vi "Gas Rack Cal UI.vi"(11 "Calling VI Ref":refnum<vi>) -> ()   [LabVIEW 2019]
uses:
  Type Defs/Units Type Def (DAQ Rack).ctl
  Type Defs/Gas Rack Channel Type Def (RIO).ctl
  Type Defs/Targets Type Def.ctl
  Type Defs/Target Cluster Type Def.ctl
  Type Defs/Setpoint Cluster Type Def.ctl
  Type Defs/Rack Version Type Def.ctl
  Type Defs/Registered System.ctl
  Type Defs/System Type.ctl
  Type Defs/TCP Data Stream Mode (PC).ctl
  <vilib>/Utility/miscctls.llb/LVRowAndColumnTypeDef.ctl
  <vilib>/Utility/file.llb/Write To Spreadsheet File (string).vi
  <vilib>/Utility/file.llb/Read From Spreadsheet File (string).vi
  <userlib>/_OpenG.lib/array/array.llb/Remove Duplicates from 1D Array (DBL)__ogtk.vi
  <userlib>/_OpenG.lib/array/array.llb/Search 1D Array (String)__ogtk.vi
  <vilib>/ptbypt/NI_PtbyPt.lvlib
  <vilib>/Analysis/NI_AALPro.lvlib
  <resource>/objmgr/daqmx.rc
  <vilib>/Utility/config.llb/NI_LVConfig.lvlib
  <vilib>/FTP/NI_FTP.lvlib
panel:
  out "RIO Found":bool
  out "Lost Connection":bool
  in  "Stop Second Loop":bool
  out "a0":dbl format="%#.4g"
  out "a2":dbl format="%#.4g"
  out "a1":dbl format="%#.4g"
  out "a3":dbl format="%#.4g"
  out "a4":dbl format="%#.4g"
  in  "App Dir":path
  in  "Load Indicator Tab":enum32{"Page 1"}(tab)
  in  "Header Tab":enum32{"Page 1", "Page 2"}(tab)
  in  "Header OK":bool
  in  "Header Cancel":bool
  in  "Header Comments":string[][](table)=[[""], [""], [""]]
  in  "Cal Standards Table":string[][](table)=[["", ""], ["", ""], ["", ""], ["", ""], ["", ""]]
  in  "Sys Cal Table":string[][](table)=[["", ""], ["", ""], ["", ""], ["", ""], ["", ""]]
  in  "Header Table 1":string[][](table)=[[""], [""], [""], [""], [""], [""], [""], [""]]
  in  "Header Table 2":string[][](table)=[[""], [""], [""], [""], [""], [""], [""]]
  in  "debug":bool=TRUE
  in  "Output Tab":enum32{"Page 1", "Page 2"}(tab)
  out "Row":i32
  in  "Main Tab":enum32{"Page 1", "Page 2"}(tab)
  in  "Channel to Cal":T1
  in  "Transfer Cal":bool
  in  "Verify Tab":enum32{"Page 1", "Page 2"}(tab)
  out "Ver Reading":dbl=0.0016 caption="reading" format="%#.4g"
  in  "Hide Devs":bool
  in  "Auto":bool
  in  "Hide Cal Values":bool
  in  "Verify Edit":bool
  in  "Verify Table":string[][](table)=[["", "0", "0"], ["", "3", "3"], ["", "6", "6"], ["", "9", "9"], ["", "12", "12"], ["", "15", "15"], ["", "", ""], ["", "", ""], ["", "", ""], ["", "", ""]]
  in  "Verify Read":bool
  in  "ms":u32=1000
  in  "avg":i32=5
  in  "Save Cal":bool
  in  "Cancel Verify":bool
  in  "Cal Tab":enum32{"Apply", "Cal"}(tab)
  in  "Cancel Cal":bool
  in  "Apply Cal":bool
  in  "Confirm Cal Point":bool
  in  "Master Value":dbl caption="cal pt" format="%#.4g"
  out "Cal Reading":dbl=0.0016 caption="reading" format="%#.4g"
  in  "4th Point Cal":bool
  out "Reading Value 4":dbl caption="reading" format="%#.4g"
  in  "Cal Value 4":dbl caption="cal pt" format="%#.4g"
  in  "5th Point Cal":bool
  out "Reading Value 5":dbl caption="reading" format="%#.4g"
  in  "Cal Value 5":dbl caption="cal pt" format="%#.4g"
  in  "Start Verification":bool
  in  "Header":bool
  out "Cal Table":string[][](table)=[["AI-00", "V", "", "", "", "", "", "", "", "", "", "", "", "", "", "", "", "", "", "", "", "", "", "", "", "", "", "", "", "", "", ""], ["AI-01", "V", "", "", "", "", "", "", "", "", "", "", "", "", "", "", "", "", "", "", "", "", "", "", "", "", "", "", "", "", "", ""], ["AI-02", "V", "", "", "", "", "", "", "", "", "", "", "", "", "", "", "", "", "", "", "", "", "", "", "", "", "", "", "", "", "", ""], ["AI-03", "V", "", "", "", "", "", "", "", "", "", "", "", "", "", "", "", "", "", "", "", "", "", "", "", "", "", "", "", "", "", ""], ["AI-04", "V", "", "", "", "", "", "", "", "", "", "", "", "", "", "", "", "", "", "", "", "", "", "", "", "", "", "", "", "", "", ""], ["AI-05", "V", "", "", "", "", "", "", "", "", "", "", "", "", "", "", "", "", "", "", "", "", "", "", "", "", "", "", "", "", "", ""], ["AI-06", "V", "", "", "", "", "", "", "", "", "", "", "", "", "", "", "", "", "", "", "", "", "", "", "", "", "", "", "", "", "", ""], ["AI-07", "V", "", "", "", "", "", "", "", "", "", "", "", "", "", "", "", "", "", "", "", "", "", "", "", "", "", "", "", "", "", ""], ["AI-08", "V", "", "", "", "", "", "", "", "", "", "", "", "", "", "", "", "", "", "", "", "", "", "", "", "", "", "", "", "", "", ""], ["AI-09", "V", "", "", "", "", "", "", "", "", "", "", "", "", "", "", "", "", "", "", "", "", "", "", "", "", "", "", "", "", "", ""], ["AI-10", "V", "", "", "", "", "", "", "", "", "", "", "", "", "", "", "", "", "", "", "", "", "", "", "", "", "", "", "", "", "", ""], ["AI-11", "V", "", "", "", "", "", "", "", "", "", "", "", "", "", "", "", "", "", "", "", "", "", "", "", "", "", "", "", "", "", ""], ["AI-12", "V", "", "", "", "", "", "", "", "", "", "", "", "", "", "", "", "", "", "", "", "", "", "", "", "", "", "", "", "", "", ""], ["AI-13", "V", "", "", "", "", "", "", "", "", "", "", "", "", "", "", "", "", "", "", "", "", "", "", "", "", "", "", "", "", "", ""], ["AI-14", "V", "", "", "", "", "", "", "", "", "", "", "", "", "", "", "", "", "", "", "", "", "", "", "", "", "", "", "", "", "", ""], ["AI-15", "V", "", "", "", "", "", "", "", "", "", "", "", "", "", "", "", "", "", "", "", "", "", "", "", "", "", "", "", "", "", ""], ["AI-16", "V", "", "", "", "", "", "", "", "", "", "", "", "", "", "", "", "", "", "", "", "", "", "", "", "", "", "", "", "", "", ""], ["AI-17", "V", "", "", "", "", "", "", "", "", "", "", "", "", "", "", "", "", "", "", "", "", "", "", "", "", "", "", "", "", "", ""], ["AI-18", "V", "", "", "", "", "", "", "", "", "", "", "", "", "", "", "", "", "", "", "", "", "", "", "", "", "", "", "", "", "", ""], ["AI-19", "V", "", "", "", "", "", "", "", "", "", "", "", "", "", "", "", "", "", "", "", "", "", "", "", "", "", "", "", "", "", ""], ["AI-20", "V", "", "", "", "", "", "", "", "", "", "", "", "", "", "", "", "", "", "", "", "", "", "", "", "", "", "", "", "", "", ""], ["AI-21", "V", "", "", "", "", "", "", "", "", "", "", "", "", "", "", "", "", "", "", "", "", "", "", "", "", "", "", "", "", "", ""], ["AI-22", "V", "", "", "", "", "", "", "", "", "", "", "", "", "", "", "", "", "", "", "", "", "", "", "", "", "", "", "", "", "", ""], ["AI-23", "V", "", "", "", "", "", "", "", "", "", "", "", "", "", "", "", "", "", "", "", "", "", "", "", "", "", "", "", "", "", ""], ["AI-24", "V", "", "", "", "", "", "", "", "", "", "", "", "", "", "", "", "", "", "", "", "", "", "", "", "", "", "", "", "", "", ""], ["AI-25", "V", "", "", "", "", "", "", "", "", "", "", "", "", "", "", "", "", "", "", "", "", "", "", "", "", "", "", "", "", "", ""], ["AI-26", "V", "", "", "", "", "", "", "", "", "", "", "", "", "", "", "", "", "", "", "", "", "", "", "", "", "", "", "", "", "", ""], ["AI-27", "V", "", "", "", "", "", "", "", "", "", "", "", "", "", "", "", "", "", "", "", "", "", "", "", "", "", "", "", "", "", ""], ["AI-28", "V", "", "", "", "", "", "", "", "", "", "", "", "", "", "", "", "", "", "", "", "", "", "", "", "", "", "", "", "", "", ""], ["AI-29", "V", "", "", "", "", "", "", "", "", "", "", "", "", "", "", "", "", "", "", "", "", "", "", "", "", "", "", "", "", "", ""], ["AI-30", "V", "", "", "", "", "", "", "", "", "", "", "", "", "", "", "", "", "", "", "", "", "", "", "", "", "", "", "", "", "", ""], ["AI-31", "V", "", "", "", "", "", "", "", "", "", "", "", "", "", "", "", "", "", "", "", "", "", "", "", "", "", "", "", "", "", ""], ["TC-00", "degF", "", "", "", "", "", "", "", "", "", "", "", "", "", "", "", "", "", "", "", "", "", "", "", "", "", "", "", "", "", ""], ["TC-01", "degF", "", "", "", "", "", "", "", "", "", "", "", "", "", "", "", "", "", "", "", "", "", "", "", "", "", "", "", "", "", ""], ["TC-02", "degF", "", "", "", "", "", "", "", "", "", "", "", "", "", "", "", "", "", "", "", "", "", "", "", "", "", "", "", "", "", ""], ["TC-03", "degF", "", "", "", "", "", "", "", "", "", "", "", "", "", "", "", "", "", "", "", "", "", "", "", "", "", "", "", "", "", ""], ["TC-04", "degF", "", "", "", "", "", "", "", "", "", "", "", "", "", "", "", "", "", "", "", "", "", "", "", "", "", "", "", "", "", ""], ["TC-05", "degF", "", "", "", "", "", "", "", "", "", "", "", "", "", "", "", "", "", "", "", "", "", "", "", "", "", "", "", "", "", ""], ["TC-06", "degF", "", "", "", "", "", "", "", "", "", "", "", "", "", "", "", "", "", "", "", "", "", "", "", "", "", "", "", "", "", ""], ["TC-07", "degF", "", "", "", "", "", "", "", "", "", "", "", "", "", "", "", "", "", "", "", "", "", "", "", "", "", "", "", "", "", ""], ["TC-08", "degF", "", "", "", "", "", "", "", "", "", "", "", "", "", "", "", "", "", "", "", "", "", "", "", "", "", "", "", "", "", ""], ["TC-09", "degF", "", "", "", "", "", "", "", "", "", "", "", "", "", "", "", "", "", "", "", "", "", "", "", "", "", "", "", "", "", ""], ["TC-10", "degF", "", "", "", "", "", "", "", "", "", "", "", "", "", "", "", "", "", "", "", "", "", "", "", "", "", "", "", "", "", ""], ["TC-11", "degF", "", "", "", "", "", "", "", "", "", "", "", "", "", "", "", "", "", "", "", "", "", "", "", "", "", "", "", "", "", ""], ["TC-12", "degF", "", "", "", "", "", "", "", "", "", "", "", "", "", "", "", "", "", "", "", "", "", "", "", "", "", "", "", "", "", ""], ["TC-13", "degF", "", "", "", "", "", "", "", "", "", "", "", "", "", "", "", "", "", "", "", "", "", "", "", "", "", "", "", "", "", ""], ["TC-14", "degF", "", "", "", "", "", "", "", "", "", "", "", "", "", "", "", "", "", "", "", "", "", "", "", "", "", "", "", "", "", ""], ["TC-15", "degF", "", "", "", "", "", "", "", "", "", "", "", "", "", "", "", "", "", "", "", "", "", "", "", "", "", "", "", "", "", ""], ["", "", "", "", "", "", "", "", "", "", "", "", "", "", "", "", "", "", "", "", "", "", "", "", "", "", "", "", "", "", "", ""]]
  out "Tank IP:":string
  in  "Start Cal":bool
  in  "1st Point Cal":bool
  out "Reading Value 1":dbl caption="Read Data" format="%#.4g"
  in  "Cal Value 1":dbl caption="Cal Point" format="%#.4g"
  in  "2nd Point Cal":bool
  out "Reading Value 2":dbl caption="reading" format="%#.4g"
  in  "Cal Value 2":dbl caption="cal pt" format="%#.4g"
  in  "Cal Unit":T2
  in  "3rd Point Cal":bool
  out "Reading Value 3":dbl caption="reading" format="%#.4g"
  in  "Cal Value 3":dbl caption="cal pt" format="%#.4g"
  in  "View Spreadsheet":bool
  # "Channel Data"
  # "System Calibration Components"
  # "Calibration Standards Used"
  # "Output Control"
  # "Enter Header Info"
  # "Calibration"
  # "Verification"
  # "Select Channel to Calibrate"
  # "Cal Spreadsheet"
  # "*Excel must be closed to return control to this app."
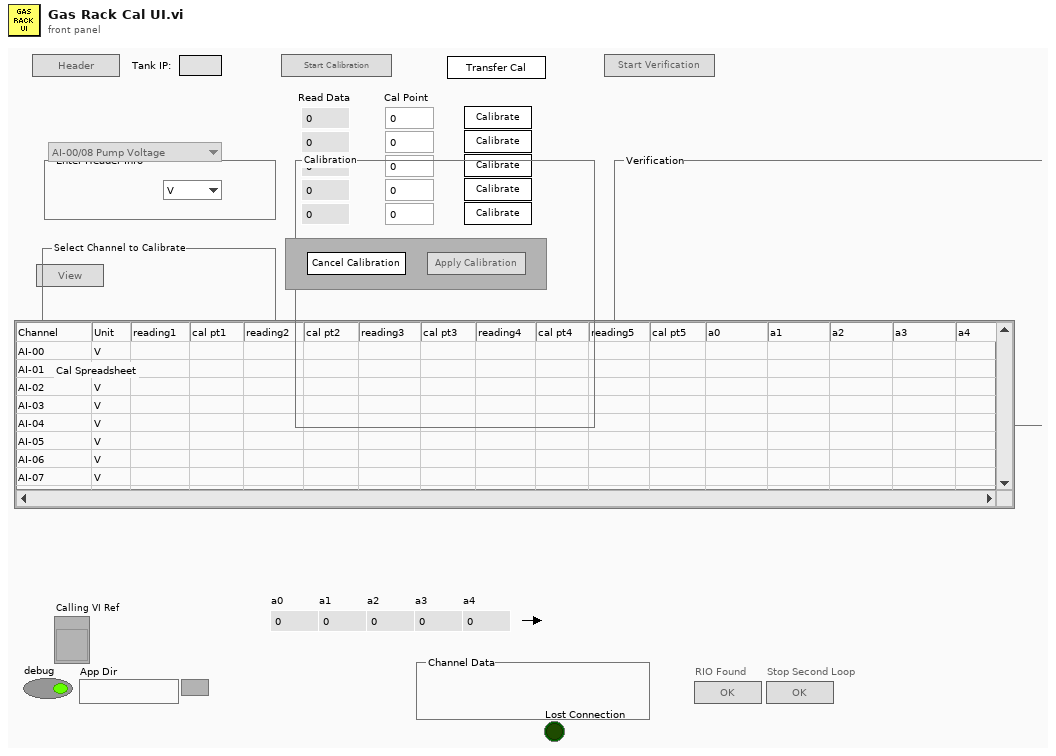
[diagram p1: front panel]
types:
  T1 = typedef "Gas Rack Channel Type Def (RIO).ctl" = enum16{"AI-00/08 Pump Voltage", "AI-01/09 Pump Current", "AI-02/10 Pressure", "AI-03/11 Flow", "AI-04/12 Controller Voltage", "AI-07/15 Controller Current", "AI-06/14 Temperature", "AI-05/13 Spare"}
  T2 = typedef "Units Type Def (DAQ Rack).ctl" = enum16{"V", "mA", "A", "Hz", "deg C"}
  T3 = typedef "Registered System.ctl" = cluster{"System Type":T4, "Serial Number":u32, "ID":string, "Cal File?":bool}
  T4 = typedef "System Type.ctl" = enum16{"DAQ Rack", "DAQ Cart", "RIO", "unknown", "open"}
  T5 = typedef "Rack Version Type Def.ctl" = enum16{"Volts & TC", "Volts", "RIO", "Volts & Current", "Cart"}
  T6 = typedef "Targets Type Def.ctl" = cluster{"V Targets":T7, "5V Targets":T7, "mA Targets":T7, "A Targets":T7, "Hz Targets":T7, "TC Targets":T7, "V Setpoints":T8, "5V Setpoints":T8, "mA Setpoints ":T8, "A Setpoints":T8, "Hz Setpoints":T8, "25A Setpoints":T8, "25A Targets":T7, "CT Targets":T7, "DegC Targets":T7, "kPa Targets":T7, "LpH Targets":T7, "CT Setpoints":T8, "DegC Setpoints":T8, "kPa Setpoints":T8, "LpH Setpoints":T8}
  T7 = typedef "Target Cluster Type Def.ctl" = cluster{"target1":dbl, "target2":dbl, "target3":dbl, "target4":dbl, "target5":dbl, "target6":dbl, "target7":dbl, "target8":dbl, "target9":dbl, "target10":dbl}
  T8 = typedef "Setpoint Cluster Type Def.ctl" = cluster{"setpoint1":dbl, "setpoint2":dbl, "setpoint3":dbl, "setpoint4":dbl, "setpoint5":dbl}
  T9 = cluster{"Error":errorcluster, "Cal Log":string[][], "Cal Log Header":string[], "Cal Files Base Path":path, "Default Cal Log":string[][], "Samples to Avg":i32, "Base Path":path, "Cal Targets Path":path, "Calling VI Ref":refnum<vi>, "Selected Chassis":tag, "debug":bool, "Verify Table":string[][], "Cal Template Path":path, "Cal Spreadsheet Path":path, "Verify Table Ref":refnum<vi>, "Init Mean":bool, "Auto":bool, "App Dir":path, "DAQ Rack":string, "Cal File Path":path, "Targets":T6, "Cal Unit":T2, "Channel to Cal":T1, "Rack Version":T5, "Verification":bool, "Registered Systems":T3[], "Desired System":T3, "Cal Target Array":string[], "LastCalPt":i32, "StreamCtrlActive":bool}
  T10 = enum8{"Enabled", "Disabled", "Disabled and Grayed Out"}
  T11 = typedef "TCP Data Stream Mode (PC).ctl" = enum16{"Init", "Read Data", "Close"}
  T12 = typedef "LVRowAndColumnTypeDef.ctl" = cluster{"Row":i32, "Column":i32}
  T13 = enum32{"Bad", "Idle", "Run top level", "Running"}
  T14 = cluster{"[0]":dbl, "[1]":dbl, "[2]":dbl, "[3]":dbl, "[4]":dbl, "[5]":dbl, "[6]":dbl, "[7]":dbl, "[8]":dbl, "[9]":dbl}
  T15 = typedef "NI_LVConfig.lvlib/Config Data RefNum.ctl" = refnum<k1>
  T16 = typedef "New Channel Type Def (RIO).ctl" = enum16{"AI-00/08 Pos 1 Pump Voltage", "AI-01/09 Pos 2 Pump Voltage", "AI-02/10 Pos 3 Pump Voltage", "AI-03/11 Pos 4 Pump Voltage", "AI-04/12 Pos 5 Pump Voltage", "AI-05/13 Pos 6 Pump Voltage", "AI-06 Spare", "AI-14 Spare", "AI-07 Spare", "AI-15 Power Supply Voltage", "AI-16 Pos 1 Pump Current", "AI-17 Pos 2 Pump Current", "AI-18 Pos 3 Pump Current", "AI-19 Pos 4 Pump Current", "AI-20 Pos 5 Pump Current", "AI-21 Pos 6 Pump Current", "AI-16 Pos 1 Pump Speed", "AI-17 Pos 2 Pump Speed", "AI-18 Pos 3 Pump Speed", "AI-19 Pos 4 Pump Speed", "AI-20 Pos 5 Pump Speed", "AI-21 Pos 6 Pump Speed", "AI-22 Pos 1 Controller Current", "AI-23 Pos 2 Controller Current", "AI-24 Pos 3 Controller Current", "AI-25 Pos 4 Controller Current", "AI-26 Pos 5 Controller Current", "AI-27 Pos 6 Controller Current", "AI-28 Tank 1 Temperature", "AI-29 Tank 2 Temperature", "AI-30 Pos 1 Pump Pressure", "AI-31 Pos 2 Pump Pressure", "AI-32 Pos 3 Pump Pressure", "AI-33 Pos 4 Pump Pressure", "AI-34 Pos 5 Pump Pressure", "AI-35 Pos 6 Pump Pressure", "AI-36 Pos 1 Pump Flow", "AI-37 Pos 2 Pump Flow", "AI-38 Pos 3 Pump Flow", "AI-39 Pos 4 Pump Flow", "AI-40 Pos 5 Pump Flow", "AI-41 Pos 6 Pump Flow", "AI-42 Spare", "AI-43 Spare", "AI-44 Spare", "AI-45 Spare", "AI-46 Spare", "AI-47 Spare", "AI-00/08 Pos 1 Controller Voltage", "AI-01/09 Pos 2 Controller Voltage", "AI-02/10 Pos 3 Controller Voltage", "AI-03/11 Pos 4 Controller Voltage", "AI-04/12 Pos 5 Controller Voltage", "AI-05/13 Pos 6 Controller Voltage"}
  T17 = cluster{"Error":errorcluster, "Cal Log":string[][], "Cal Log Header":string[], "Cal Files Base Path":path, "Default Cal Log":string[][], "Samples to Avg":i32, "Base Path":path, "Cal Targets Path":path, "Calling VI Ref":refnum<vi>, "Selected Chassis":tag, "debug":bool, "Verify Table":string[][], "Cal Template Path":path, "Cal Spreadsheet Path":path, "Verify Table Ref":refnum<vi>, "Init Mean":bool, "Auto":bool, "App Dir":path, "DAQ Rack":string, "Cal File Path":path, "Targets":T6, "Cal Unit":T2, "Channel to Cal":T16, "Rack Version":T5, "Verification":bool, "Registered Systems":T3[], "Desired System":T3, "Cal Target Array":string[], "LastCalPt":i32}
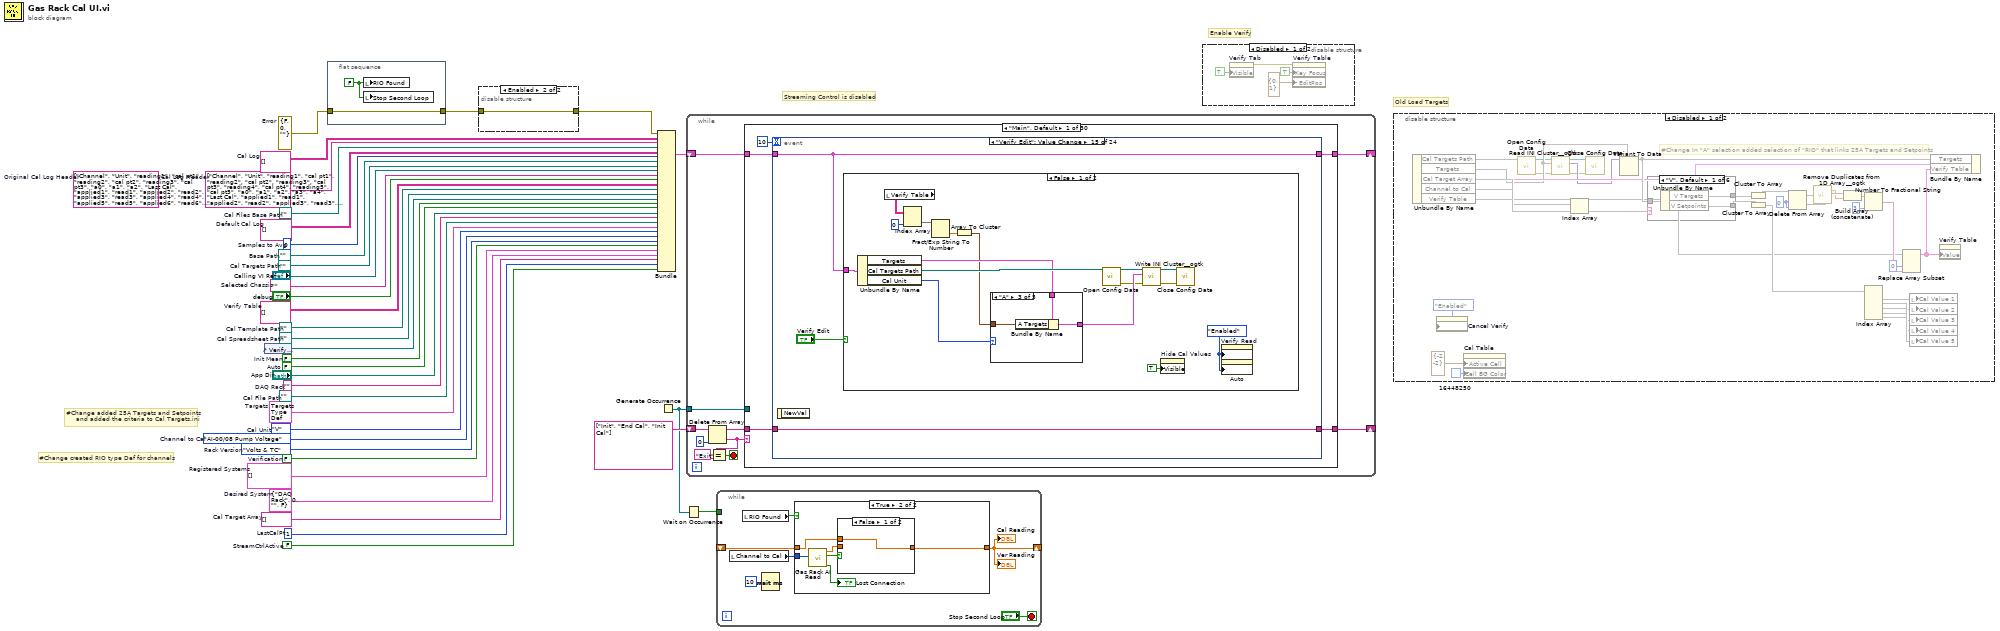
[diagram p0: block diagram]
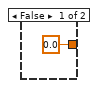
[diagram p2: hidden frame]
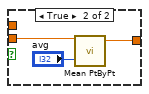
[diagram p3: hidden frame]
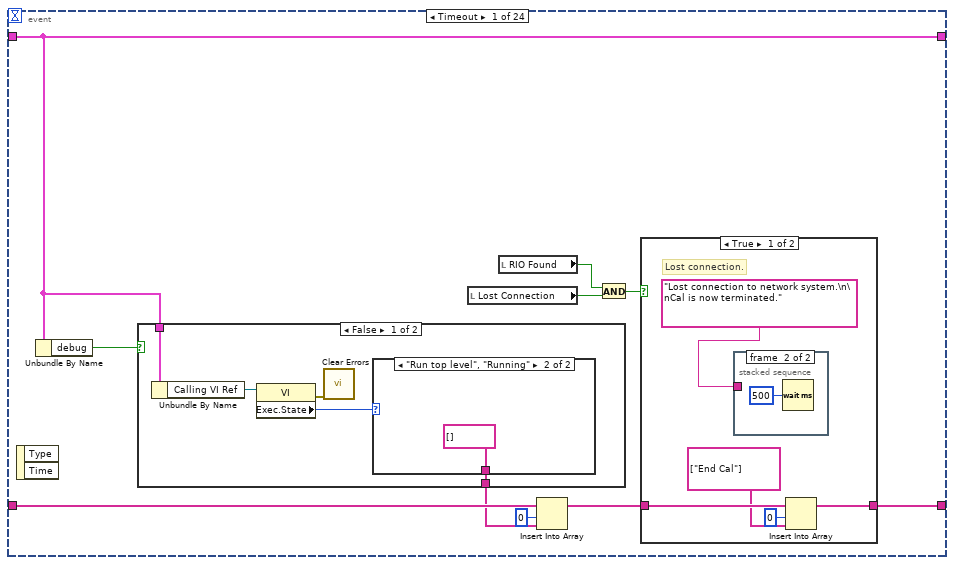
[diagram p4: hidden frame]
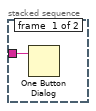
[diagram p5: hidden frame]
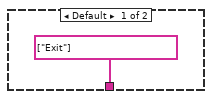
[diagram p7: hidden frame]
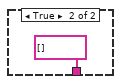
[diagram p8: hidden frame]
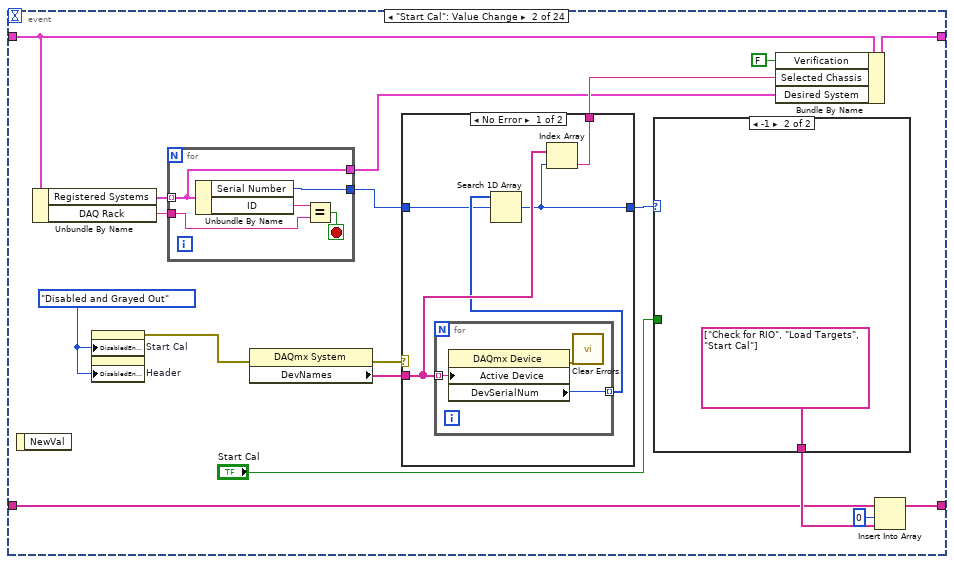
[diagram p9: hidden frame]
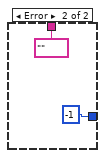
[diagram p10: hidden frame]
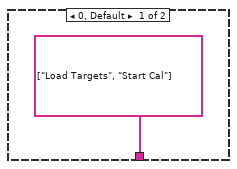
[diagram p11: hidden frame]
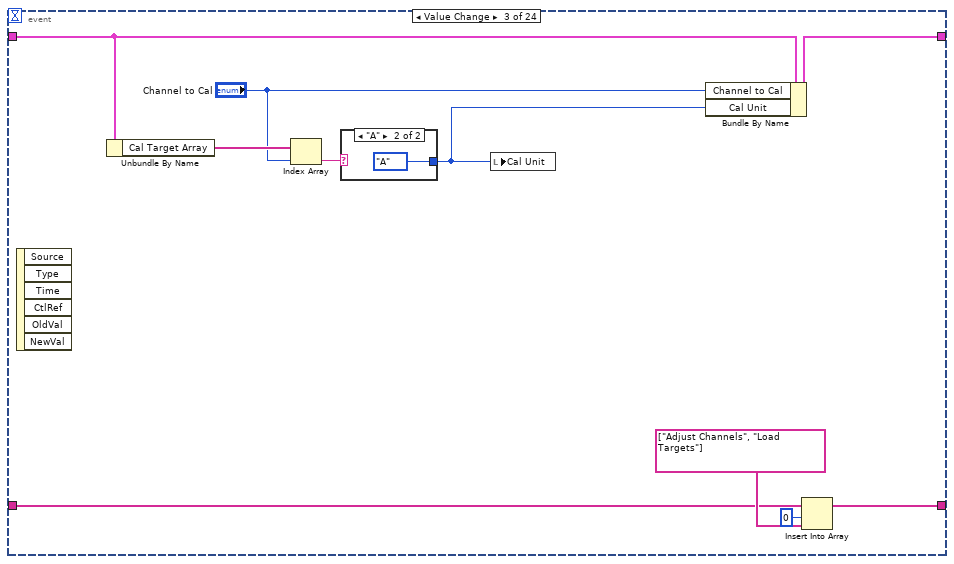
[diagram p12: hidden frame]
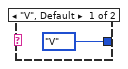
[diagram p13: hidden frame]
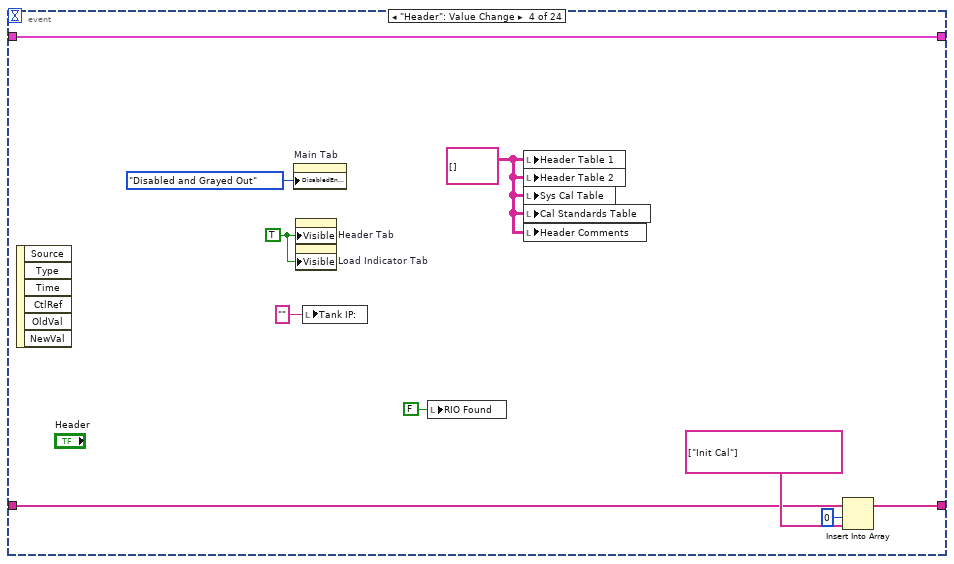
[diagram p14: hidden frame]
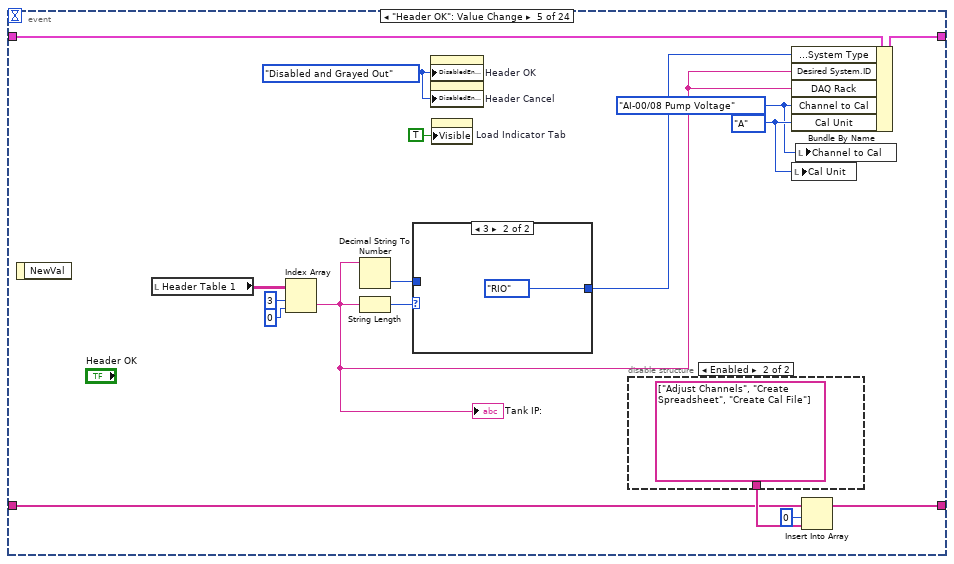
[diagram p15: hidden frame]
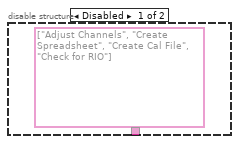
[diagram p16: hidden frame]
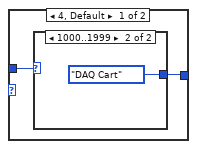
[diagram p17: hidden frame]
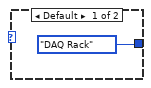
[diagram p18: hidden frame]
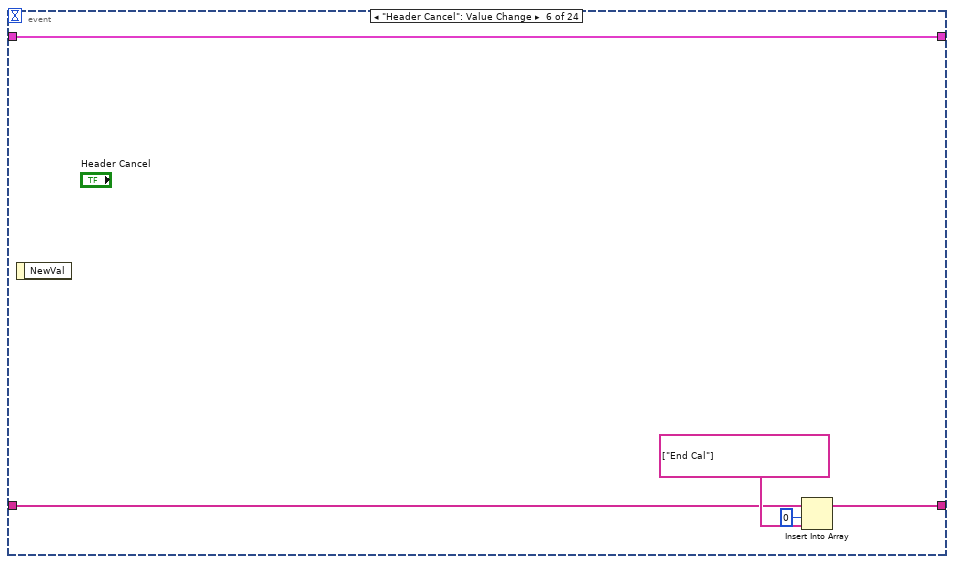
[diagram p19: hidden frame]
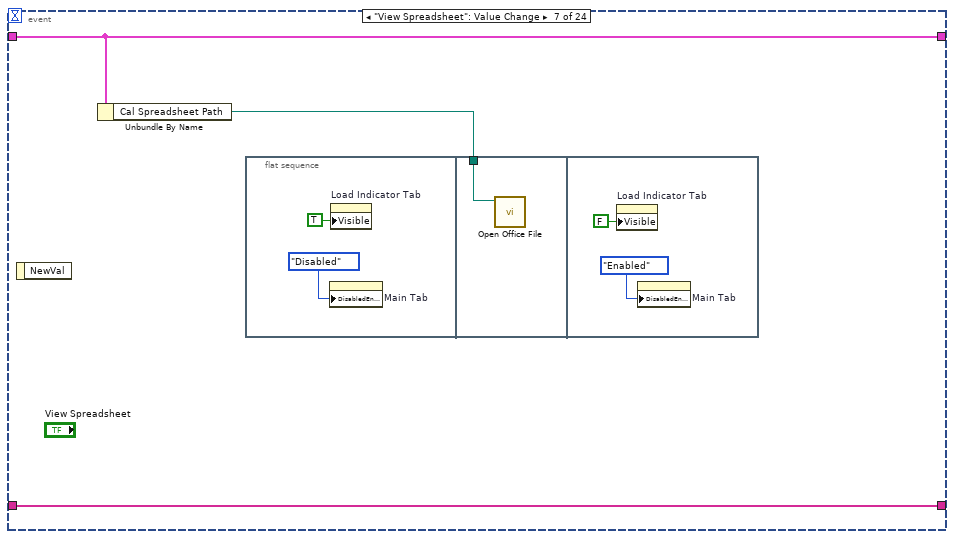
[diagram p20: hidden frame]
diagram:
  w1 = Gas_Rack_Channel_Type_Def_(RIO)."AI-00/08 Pump Voltage"  # Channel to Cal
  w8 = FALSE  # StreamCtrlActive
  w9 = 1  # LastCalPt
  w11 = string[] ["Channel", "Unit", "reading1", "cal pt1", "reading2", "cal pt2", "reading3", "cal pt3", "reading4", "cal pt4", "reading5", "cal pt5", "a0", "a1", "a2", "a3", "a4", "Last Cal", "applied1", "read1", "applied2", "read2", "applied3", "read3", "applied4", "read4", "applied5", "read5", "applied6", "read6", "applied7", "read7", "applied8", "read8", "applied9", "read9", "applied10", "read10"]  # Cal Log Header
  w12 = string[] []  # Cal Target Array
  w13 = T3 {"System Type"=enum."DAQ Rack", "Serial Number"=0, "ID"="", "Cal File?"=FALSE}  # Desired System
  w14 = T3[] []  # Registered Systems
  w15 = FALSE  # Verification
  w16 = Rack_Version_Type_Def."Volts & TC"  # Rack Version
  w17 = Units_Type_Def_(DAQ_Rack)."V"  # Cal Unit
  w18 = T6 {"V Targets"={"target1"=0.0, "target2"=0.0, "target3"=0.0, "target4"=0.0, "target5"=0.0, "target6"=0.0, "target7"=0.0, "target8"=0.0, "target9"=0.0, "target10"=0.0}, "5V Targets"={"target1"=0.0, "target2"=0.0, "target3"=0.0, "target4"=0.0, "target5"=0.0, "target6"=0.0, "target7"=0.0, "target8"=0.0, "target9"=0.0, "target10"=0.0}, "mA Targets"={"target1"=0.0, "target2"=0.0, "target3"=0.0, "target4"=0.0, "target5"=0.0, "target6"=0.0, "target7"=0.0, "target8"=0.0, "target9"=1.0, "target10"=0.0}, "A Targets"={"target1"=0.0, "target2"=0.0, "target3"=0.0, "target4"=0.0, "target5"=0.0, "target6"=0.0, "target7"=0.0, "target8"=0.0, "target9"=0.0, "target10"=0.0}, "Hz Targets"={"target1"=0.0, "target2"=0.0, "target3"=0.0, "target4"=0.0, "target5"=0.0, "target6"=0.0, "target7"=0.0, "target8"=0.0, "target9"=0.0, "target10"=0.0}, "TC Targets"={"target1"=0.0, "target2"=0.0, "target3"=0.0, "target4"=0.0, "target5"=0.0, "target6"=0.0, "target7"=0.0, "target8"=0.0, "target9"=0.0, "target10"=0.0}, "V Setpoints"={"setpoint1"=0.0, "setpoint2"=0.0, "setpoint3"=0.0, "setpoint4"=0.0, "setpoint5"=0.0}, "5V Setpoints"={"setpoint1"=0.0, "setpoint2"=0.0, "setpoint3"=0.0, "setpoint4"=0.0, "setpoint5"=0.0}, "mA Setpoints "={"setpoint1"=0.0, "setpoint2"=0.0, "setpoint3"=0.0, "setpoint4"=0.0, "setpoint5"=0.0}, "A Setpoints"={"setpoint1"=0.0, "setpoint2"=0.0, "setpoint3"=0.0, "setpoint4"=0.0, "setpoint5"=0.0}, "Hz Setpoints"={"setpoint1"=0.0, "setpoint2"=0.0, "setpoint3"=0.0, "setpoint4"=0.0, "setpoint5"=0.0}, "25A Setpoints"={"setpoint1"=0.0, "setpoint2"=0.0, "setpoint3"=0.0, "setpoint4"=0.0, "setpoint5"=0.0}, "25A Targets"={"target1"=0.0, "target2"=0.0, "target3"=0.0, "target4"=0.0, "target5"=0.0, "target6"=0.0, "target7"=0.0, "target8"=0.0, "target9"=0.0, "target10"=0.0}, "CT Targets"={"target1"=0.0, "target2"=0.0, "target3"=0.0, "target4"=0.0, "target5"=0.0, "target6"=0.0, "target7"=0.0, "target8"=0.0, "target9"=0.0, "target10"=0.0}, "DegC Targets"={"target1"=0.0, "target2"=0.0, "target3"=0.0, "target4"=0.0, "target5"=0.0, "target6"=0.0, "target7"=0.0, "target8"=0.0, "target9"=0.0, "target10"=0.0}, "kPa Targets"={"target1"=0.0, "target2"=0.0, "target3"=0.0, "target4"=0.0, "target5"=0.0, "target6"=0.0, "target7"=0.0, "target8"=0.0, "target9"=0.0, "target10"=0.0}, "LpH Targets"={"target1"=0.0, "target2"=0.0, "target3"=0.0, "target4"=0.0, "target5"=0.0, "target6"=0.0, "target7"=0.0, "target8"=0.0, "target9"=0.0, "target10"=0.0}, "CT Setpoints"={"setpoint1"=0.0, "setpoint2"=0.0, "setpoint3"=0.0, "setpoint4"=0.0, "setpoint5"=0.0}, "DegC Setpoints"={"setpoint1"=0.0, "setpoint2"=0.0, "setpoint3"=0.0, "setpoint4"=0.0, "setpoint5"=0.0}, "kPa Setpoints"={"setpoint1"=0.0, "setpoint2"=0.0, "setpoint3"=0.0, "setpoint4"=0.0, "setpoint5"=0.0}, "LpH Setpoints"={"setpoint1"=0.0, "setpoint2"=0.0, "setpoint3"=0.0, "setpoint4"=0.0, "setpoint5"=0.0}}  # Targets
  w19 = path ""  # Cal File Path
  w20 = ""  # DAQ Rack
  w22 = FALSE  # Auto
  w23 = FALSE  # Init Mean
  w25 = path ""  # Cal Spreadsheet Path
  w26 = path ""  # Cal Template Path
  w27 = string[][] []  # Verify Table
  w29 = tag ""  # Selected Chassis
  w31 = path ""  # Cal Targets Path
  w32 = path ""  # Base Path
  w33 = 0  # Samples to Avg
  w34 = string[][] []  # Default Cal Log
  w35 = path ""  # Cal Files Base Path
  (unwired) string[] ["Channel", "Unit", "reading1", "cal pt1", "reading2", "cal pt2", "reading3", "cal pt3", "a0", "a1", "a2", "Last Cal", "applied1", "read1", "applied2", "read2", "applied3", "read3", "applied4", "read4", "applied5", "read5", "applied6", "read6", "applied7", "read7", "applied8", "read8", "applied9", "read9", "applied10", "read10"]  # Original Cal Log Header
  w36 = string[][] []  # Cal Log
  w10 = errorcluster {"status"=FALSE, "code"=0, "source"=""}  # Error
  # "Old Load Targets"
  # "Streaming Control is disabled"
  # "Enable Verify"
  # "#Change created RIO type Def for channels"
  # "#Change added 25A Targets and Setpoints\n     and added the criteria to Cal Targets.ini"
  n1 = control-ref of="Verify Table Ref"() -> (w24:refnum<vi>)
  n2 = flat-sequence {
    tunnel: w10 -> [w38]
    tunnel: [w38] -> w7
    frame #0 {
      w37 = FALSE ("RIO Found")
      n3 = local write "RIO Found"(w37) -> ()
      n4 = local write "Stop Second Loop"(w37) -> ()
    }
  }
  n5 = disable-structure shown="Enabled" {
    disable-tunnel: w7 -> [w42 w43]
    disable-tunnel: [w40 w43] -> w6
    frame Disabled {
      w39 = TRUE ("Visible")
      n6 = property on="Cal Tab" class="TabCtl (strict)"(error in=w42, "Visible"=w39) -> (error out=w41:errorcluster)  [unwired: 1 in, 1 out]
      n7 = property on="Verify Tab" class="TabCtl (strict)"(error in=w41, "Visible"=w39) -> (error out=w40:errorcluster)  [unwired: 1 in, 1 out]
    }
    frame Enabled {
    }
  }
  n8 = Bundle("Error"=w6, "Cal Log"=w36, "Cal Log Header"=w11, "Cal Files Base Path"=w35, "Default Cal Log"=w34, "Samples to Avg"=w33, "Base Path"=w32, "Cal Targets Path"=w31, "Calling VI Ref"="Calling VI Ref", "Selected Chassis"=w29, "debug"="debug", "Verify Table"=w27, "Cal Template Path"=w26, "Cal Spreadsheet Path"=w25, "Verify Table Ref"=w24, "Init Mean"=w23, "Auto"=w22, "App Dir"="App Dir", "DAQ Rack"=w20, "Cal File Path"=w19, "Targets"=w18, "Cal Unit"=w17, "Channel to Cal"=w1, "Rack Version"=w16, "Verification"=w15, "Registered Systems"=w14, "Desired System"=w13, "Cal Target Array"=w12, "LastCalPt"=w9, "StreamCtrlActive"=w8) -> (w4:T9)  [unwired: 1 in]
  n9 = Generate Occurrence() -> (w3:refnum<k4>)
  n10 = Wait on Occurrence(2:w3) -> (0:w2:bool)  [unwired: 2 in]
  n11 = while {
    shift-right: [w46] -> _
    shift-left: string[] ["Init", "End Cal", "Init Cal"] -> [w53]
    shift-right: [w48] -> _
    shift-left: w4 -> [w49]
    tunnel: w3 -> [w44]
    stop <- w52 stop-if-true
    n12 = Delete From Array(array=w53, index=0) -> (deleted portion=w45:string, array with subset deleted=w51:string[])  [unwired: 1 in]
    n13 = Equal?(x=w45, y="Exit" ("x")) -> (x = y?=w52:bool)
    n14 = case shown="\"Main\", Default" w45 {
      selector: w45 -> [_ _ _ _ _ _ _ _ _ _ _ _ _ _ _ w852 _ _ _ _ _ _ _ _ _ _ _ _ _ _]
      tunnel: w51 -> [w57 w425 w440 w448 w465 w514 w544 w547 w551 w582 w611 w640 w664 w722 w842 w854 w868 w884 w968 w995 w1005 w1068 w1146 w1169 w1186 w1197 w1220 w1233 w1241 w1244]
      tunnel: w49 -> [w56 w418 w441 w454 w462 w513 w543 w546 w549 w585 w613 w634 w662 w770 w845 w849 w869 w878 w954 w979 w1006 w1029 w1107 w1168 w1184 w1195 w1217 w1223 w1239 w1243]
      tunnel: [w55 w402 w441 w453 w462 w512 w542 w546 w549 w584 w613 w633 w666 w779 w845 w848 w869 w878 w954 w974 w1006 w1029 w1107 w1168 w1183 w1195 w1217 w1223 w1240 w1243] -> w48
      tunnel: [w54 w425 w440 w445 w464 w514 w544 w547 w550 w583 w612 w641 w665 w721 w842 w854 w868 w885 w967 w996 w1005 w1069 w1147 w1169 w1185 w1196 w1220 w1234 w1241 w1244] -> w46
      tunnel: w44 -> [_ w401 _ _ _ _ _ _ _ _ _ _ _ _ _ _ _ _ _ _ _ _ _ _ _ _ _ _ _ _]
      frame "Main", Default {
        n15 = event shown="[14] \"Verify Edit\": Value Change" {
          selector: _ -> [_ _ _ _ _ _ _ _ _ _ _ _ _ _ _ _ _ _ _ _ _ _ _ _]
          dyn-events: _ -> [_ _ _ _ _ _ _ _ _ _ _ _ _ _ _ _ _ _ _ _ _ _ _ _]
          timeout: 10 -> [_ _ _ _ _ _ _ _ _ _ _ _ _ _ _ _ _ _ _ _ _ _ _ _]
          tunnel: w57 -> [w68 w100 w126 w136 w154 w169 w173 _ _ _ _ _ _ w232 w257 _ w300 _ w319 w352 w358 w382 w389 w395]
          tunnel: [w66 w96 w129 w141 w148 w167 w171 w186 w194 w202 w210 w218 w221 w235 w259 w294 w298 w307 w320 w353 w356 w375 w391 w396] -> w55
          tunnel: w56 -> [w66 w97 w124 w141 w149 w167 w171 w186 w194 w202 w210 w218 w221 w237 w259 w294 w299 w308 w320 w353 w356 w375 w391 w397]
          tunnel: [w61 w101 w125 w135 w155 w168 w173 w183 w191 w199 w207 w215 string[] ["Stop Verification"] w233 w257 string[] ["Save Cal"] w300 string[] ["Calc Dev", "Cal Review"] w319 w351 w357 w382 w390 w395] -> w54
          event Timeout {
            n16 = event-data() -> ()  [unwired: 1 in, 2 out]
            n17 = Unbundle By Name(w66) -> ("debug"=w65:bool)
            n18 = case shown="False" w65 {
              tunnel: [w81 string[] []] -> w67
              tunnel: w66 -> [w78 _]
              frame False {
                n19 = Unbundle By Name(w78) -> ("Calling VI Ref"=w80:refnum<vi>)
                n20 = property class="VI"(reference=w80) -> (error out=w77:errorcluster, "Exec.State"=w79:T13)  [unwired: 1 in, 1 out]
                n21 = call <vilib>:"Clear Errors.vi"("error in (no error)"=w77) -> ()  [unwired: 5 in, 2 out]
                n22 = case shown="\"Run top level\", \"Running\"" w79 {
                  tunnel: [string[] ["Exit"] string[] []] -> w81
                  frame Default {
                  }
                  frame "Run top level", "Running" {
                  }
                }
              }
              frame True {
              }
            }
            n23 = local read "Lost Connection"() -> (w60:bool)
            n24 = local read "RIO Found"() -> (w63:bool)
            n25 = Insert Into Array(array=w68, index=0, new element=w67) -> (w62:string[])
            n26 = And(x=w63, y=w60) -> (x .and. y?=w59:bool)
            n27 = case shown="True" w59 {
              tunnel: w62 -> [w73 w76]
              tunnel: [w70 w76] -> w61
              frame True {
                # "Lost connection."
                n28 = stacked-sequence {
                  tunnel: "Lost connection to network system.\n\nCal is now terminated." ("message") -> [w74 _]
                  frame #0 {
                    n29 = One Button Dialog(message=w74) -> ()  [unwired: 1 in, 1 out]
                  }
                  frame #1 {
                    n30 = Wait (ms)(milliseconds to wait=u32 500) -> ()  [unwired: 1 out]
                  }
                }
                n31 = Insert Into Array(array=w73, index=0, new element=string[] ["End Cal"]) -> (w70:string[])
              }
              frame False {
                # "Or not yet connected"
                # "Still connected."
              }
            }
          }
          event "Start Cal": Value Change {
            w92 = T10."Disabled and Grayed Out" ("Disabled")
            n32 = event-data() -> ()  [unwired: 1 in, 1 out]
            n33 = Unbundle By Name(w97) -> ("Registered Systems"=w89:T3[], "DAQ Rack"=w88:string)
            n34 = property on="Start Cal" class="Bool"("DisabledEnum"=w92) -> (error out=w91:errorcluster)  [unwired: 2 in, 1 out]
            n35 = property on="Header" class="Bool"("DisabledEnum"=w92) -> ()  [unwired: 2 in, 2 out]
            n36 = for {
              tunnel: w89 -> [w103] mode=indexing
              tunnel: w88 -> [w106]
              tunnel: [w104] -> w87
              tunnel: [w103] -> w86
              stop <- w105 stop-if-true
              n37 = Unbundle By Name(w103) -> ("Serial Number"=w104:u32, "ID"=w107:string)
              n38 = Equal?(x=w107, y=w106) -> (x = y?=w105:bool)
            }
            n39 = property class="DAQmx System"(error in=w91) -> (error out=w94:errorcluster, "DevNames"=w99:tag[])  [unwired: 1 in, 1 out]
            n40 = case shown="No Error" w94 {
              tunnel: w87 -> [w108 _]
              tunnel: w99 -> [w112 _]
              tunnel: [w111 -1 ("index of element")] -> w98
              tunnel: [w110 tag ""] -> w95
              frame No Error {
                n41 = for {
                  tunnel: w112 -> [w115] mode=indexing
                  tunnel: [w114] -> w109 mode=indexing
                  n42 = property class="DAQmx Device"("Active Device"=w115) -> (error out=w113:errorcluster, "DevSerialNum"=w114:u32)  [unwired: 2 in, 1 out]
                  n43 = call <vilib>:"Clear Errors.vi"("error in (no error)"=w113) -> ()  [unwired: 5 in, 2 out]
                }
                n44 = Search 1D Array(1D array=w109, element=w108) -> (index of element=w111:i32)  [unwired: 1 in]
                n45 = Index Array(array=w112, index=w111) -> (element=w110:tag)
              }
              frame Error {
              }
            }
            n46 = case shown="-1" w98 {
              tunnel: [string[] ["Load Targets", "Start Cal"] string[] ["Check for RIO", "Load Targets", "Start Cal"]] -> w102
              tunnel: "Start Cal" -> [_ _]
              frame 0, Default {
              }
              frame -1 {
              }
            }
            n47 = Bundle By Name(cluster=w97, "Verification"=FALSE, "Selected Chassis"=w95, "Desired System"=w86) -> (w96:T9)
            n48 = Insert Into Array(array=w100, index=0, new element=w102) -> (w101:string[])
          }
          event Value Change {
            n49 = event-data() -> ()  [unwired: 1 in, 6 out]
            n50 = Unbundle By Name(w124) -> ("Cal Target Array"=w123:string[])
            n51 = Index Array(array=w123, index="Channel to Cal") -> (element=w122:string)
            n52 = case shown="\"A\"" w122 {
              tunnel: [Units_Type_Def_(DAQ_Rack)."V" ("Cal Unit") Units_Type_Def_(DAQ_Rack)."A" ("Cal Unit")] -> w121
              frame "V", Default {
              }
              frame "A" {
              }
            }
            n53 = local write "Cal Unit"(w121) -> ()
            n54 = Bundle By Name(cluster=w124, "Channel to Cal"="Channel to Cal", "Cal Unit"=w121) -> (w129:T9)
            n55 = Insert Into Array(array=w126, index=0, new element=string[] ["Adjust Channels", "Load Targets"]) -> (w125:string[])
          }
          event "Header": Value Change {
            w139 = string[][] [] ("Header Table 1")
            w138 = TRUE ("Visible")
            n56 = event-data() -> ()  [unwired: 1 in, 6 out]
            n57 = property on="Main Tab" class="TabCtl (strict)"("DisabledEnum"=T10."Disabled and Grayed Out" ("Disabled")) -> ()  [unwired: 2 in, 2 out]
            n58 = property on="Header Tab" class="TabCtl (strict)"("Visible"=w138) -> ()  [unwired: 2 in, 2 out]
            n59 = property on="Load Indicator Tab" class="TabCtl (strict)"("Visible"=w138) -> ()  [unwired: 2 in, 2 out]
            n60 = local write "Tank IP:"("" ("DAQ Rack")) -> ()
            n61 = local write "RIO Found"(FALSE ("RIO Found")) -> ()
            n62 = local write "Header Table 1"(w139) -> ()
            n63 = local write "Header Table 2"(w139) -> ()
            n64 = local write "Sys Cal Table"(w139) -> ()
            n65 = local write "Cal Standards Table"(w139) -> ()
            n66 = local write "Header Comments"(w139) -> ()
            n67 = Insert Into Array(array=w136, index=0, new element=string[] ["Init Cal"]) -> (w135:string[])
          }
          event "Header OK": Value Change {
            w142 = Gas_Rack_Channel_Type_Def_(RIO)."AI-00/08 Pump Voltage" ("Channel to Cal")
            w147 = Units_Type_Def_(DAQ_Rack)."A" ("Cal Unit")
            w158 = T10."Disabled and Grayed Out" ("Disabled")
            n68 = event-data() -> ()  [unwired: 1 in, 1 out]
            n69 = local read "Header Table 1"() -> (w152:string[][])
            n70 = Index Array(array=w152, index (row)=3, index (col)=0 ("disabled index (col)")) -> (element=w144:string)
            "Tank IP:" <- w144
            n71 = Decimal String To Number(string=w144) -> (number=w143:i32)  [unwired: 2 in, 1 out]
            n72 = String Length(string=w144) -> (length=w146:i32)
            n73 = case shown="3" w146 {
              tunnel: [w161 System_Type."RIO" ("Desired System.System Type")] -> w145
              tunnel: w143 -> [w162 _]
              frame 4, Default {
                n74 = case shown="1000..1999" w162 {
                  tunnel: [System_Type."DAQ Rack" ("Desired System.System Type") System_Type."DAQ Cart" ("Desired System.System Type")] -> w161
                  frame Default {
                  }
                  frame 1000..1999 {
                  }
                }
              }
              frame 3 {
              }
            }
            n75 = property on="Header OK" class="Bool"("DisabledEnum"=w158) -> ()  [unwired: 2 in, 2 out]
            n76 = property on="Header Cancel" class="Bool"("DisabledEnum"=w158) -> ()  [unwired: 2 in, 2 out]
            n77 = property on="Load Indicator Tab" class="TabCtl (strict)"("Visible"=TRUE) -> ()  [unwired: 2 in, 2 out]
            n78 = disable-structure shown="Enabled" {
              disable-tunnel: [string[] ["Adjust Channels", "Create Spreadsheet", "Create Cal File", "Check for RIO"] string[] ["Adjust Channels", "Create Spreadsheet", "Create Cal File"]] -> w156
              frame Disabled {
              }
              frame Enabled {
              }
            }
            n79 = Bundle By Name(cluster=w149, "Desired System.System Type"=w145, "Desired System.ID"=w144, "DAQ Rack"=w144, "Channel to Cal"=w142, "Cal Unit"=w147) -> (w148:T9)
            n80 = local write "Cal Unit"(w147) -> ()
            n81 = local write "Channel to Cal"(w142) -> ()
            n82 = Insert Into Array(array=w154, index=0, new element=w156) -> (w155:string[])
          }
          event "Header Cancel": Value Change {
            n83 = event-data() -> ()  [unwired: 1 in, 1 out]
            n84 = Insert Into Array(array=w169, index=0, new element=string[] ["End Cal"]) -> (w168:string[])
          }
          event "View Spreadsheet": Value Change {
            n85 = event-data() -> ()  [unwired: 1 in, 1 out]
            n86 = Unbundle By Name(w171) -> ("Cal Spreadsheet Path"=w172:path)
            n87 = flat-sequence {
              tunnel: w172 -> [w176]
              frame #0 {
                n88 = property on="Main Tab" class="TabCtl (strict)"("DisabledEnum"=T10."Disabled" ("Disabled")) -> ()  [unwired: 2 in, 2 out]
                n89 = property on="Load Indicator Tab" class="TabCtl (strict)"("Visible"=TRUE) -> ()  [unwired: 2 in, 2 out]
              }
              frame #1 {
                n90 = call "Open Office File.vi"("Selection a Word (.doc, .docx), Excel (.xls, .xlsx), or Powerpoint (.ppt, .pptx) Document..."=w176) -> ()  [unwired: 10 in, 1 out]
              }
              frame #2 {
                n91 = property on="Load Indicator Tab" class="TabCtl (strict)"("Visible"=FALSE) -> ()  [unwired: 2 in, 2 out]
                n92 = property on="Main Tab" class="TabCtl (strict)"("DisabledEnum"=T10."Enabled" ("Disabled")) -> ()  [unwired: 2 in, 2 out]
              }
            }
          }
          event "1st Point Cal": Value Change {
            n93 = event-data() -> ()  [unwired: 1 in, 1 out]
            n94 = Select(t=T10."Disabled" ("Disabled"), s="1st Point Cal", f=T10."Enabled" ("Disabled")) -> (s? t:f=w182:T10)
            n95 = property on="Cal Value 1" class="DigNum (strict)"("DisabledEnum"=w182) -> ()  [unwired: 2 in, 2 out]
            n96 = property on="Cal Value 2" class="DigNum (strict)"("DisabledEnum"=w182) -> ()  [unwired: 2 in, 2 out]
            n97 = property on="Cal Value 3" class="DigNum (strict)"("DisabledEnum"=w182) -> ()  [unwired: 2 in, 2 out]
            n98 = property on="Cal Value 4" class="DigNum (strict)"("DisabledEnum"=w182) -> ()  [unwired: 2 in, 2 out]
            n99 = property on="Cal Value 5" class="DigNum (strict)"("DisabledEnum"=w182) -> ()  [unwired: 2 in, 2 out]
            n100 = property on="2nd Point Cal" class="Bool (strict)"("DisabledEnum"=w182) -> ()  [unwired: 2 in, 2 out]
            n101 = property on="3rd Point Cal" class="Bool (strict)"("DisabledEnum"=w182) -> ()  [unwired: 2 in, 2 out]
            n102 = property on="4th Point Cal" class="Bool (strict)"("DisabledEnum"=w182) -> ()  [unwired: 2 in, 2 out]
            n103 = property on="5th Point Cal" class="Bool (strict)"("DisabledEnum"=w182) -> ()  [unwired: 2 in, 2 out]
            n104 = Select(t=string[] ["Calibrating 1"], s="1st Point Cal", f=string[] ["Stop Calibrating"]) -> (s? t:f=w183:string[])
          }
          event "2nd Point Cal": Value Change {
            n105 = event-data() -> ()  [unwired: 1 in, 1 out]
            n106 = Select(t=T10."Disabled" ("Disabled"), s="2nd Point Cal", f=T10."Enabled" ("Disabled")) -> (s? t:f=w190:T10)
            n107 = property on="Cal Value 1" class="DigNum (strict)"("DisabledEnum"=w190) -> ()  [unwired: 2 in, 2 out]
            n108 = property on="Cal Value 2" class="DigNum (strict)"("DisabledEnum"=w190) -> ()  [unwired: 2 in, 2 out]
            n109 = property on="Cal Value 3" class="DigNum (strict)"("DisabledEnum"=w190) -> ()  [unwired: 2 in, 2 out]
            n110 = property on="Cal Value 4" class="DigNum (strict)"("DisabledEnum"=w190) -> ()  [unwired: 2 in, 2 out]
            n111 = property on="Cal Value 5" class="DigNum (strict)"("DisabledEnum"=w190) -> ()  [unwired: 2 in, 2 out]
            n112 = property on="1st Point Cal" class="Bool (strict)"("DisabledEnum"=w190) -> ()  [unwired: 2 in, 2 out]
            n113 = property on="3rd Point Cal" class="Bool (strict)"("DisabledEnum"=w190) -> ()  [unwired: 2 in, 2 out]
            n114 = property on="4th Point Cal" class="Bool (strict)"("DisabledEnum"=w190) -> ()  [unwired: 2 in, 2 out]
            n115 = property on="5th Point Cal" class="Bool (strict)"("DisabledEnum"=w190) -> ()  [unwired: 2 in, 2 out]
            n116 = Select(t=string[] ["Calibrating 2"], s="2nd Point Cal", f=string[] ["Stop Calibrating"]) -> (s? t:f=w191:string[])
          }
          event "3rd Point Cal": Value Change {
            n117 = event-data() -> ()  [unwired: 1 in, 1 out]
            n118 = Select(t=T10."Disabled" ("Disabled"), s="3rd Point Cal", f=T10."Enabled" ("Disabled")) -> (s? t:f=w198:T10)
            n119 = property on="Cal Value 1" class="DigNum (strict)"("DisabledEnum"=w198) -> ()  [unwired: 2 in, 2 out]
            n120 = property on="Cal Value 2" class="DigNum (strict)"("DisabledEnum"=w198) -> ()  [unwired: 2 in, 2 out]
            n121 = property on="Cal Value 3" class="DigNum (strict)"("DisabledEnum"=w198) -> ()  [unwired: 2 in, 2 out]
            n122 = property on="Cal Value 4" class="DigNum (strict)"("DisabledEnum"=w198) -> ()  [unwired: 2 in, 2 out]
            n123 = property on="Cal Value 5" class="DigNum (strict)"("DisabledEnum"=w198) -> ()  [unwired: 2 in, 2 out]
            n124 = property on="1st Point Cal" class="Bool (strict)"("DisabledEnum"=w198) -> ()  [unwired: 2 in, 2 out]
            n125 = property on="2nd Point Cal" class="Bool (strict)"("DisabledEnum"=w198) -> ()  [unwired: 2 in, 2 out]
            n126 = property on="4th Point Cal" class="Bool (strict)"("DisabledEnum"=w198) -> ()  [unwired: 2 in, 2 out]
            n127 = property on="5th Point Cal" class="Bool (strict)"("DisabledEnum"=w198) -> ()  [unwired: 2 in, 2 out]
            n128 = Select(t=string[] ["Calibrating 3"], s="3rd Point Cal", f=string[] ["Stop Calibrating"]) -> (s? t:f=w199:string[])
          }
          event "4th Point Cal": Value Change {
            n129 = event-data() -> ()  [unwired: 1 in, 6 out]
            n130 = Select(t=T10."Disabled" ("Disabled"), s="4th Point Cal", f=T10."Enabled" ("Disabled")) -> (s? t:f=w206:T10)
            n131 = property on="Cal Value 1" class="DigNum (strict)"("DisabledEnum"=w206) -> ()  [unwired: 2 in, 2 out]
            n132 = property on="Cal Value 2" class="DigNum (strict)"("DisabledEnum"=w206) -> ()  [unwired: 2 in, 2 out]
            n133 = property on="Cal Value 3" class="DigNum (strict)"("DisabledEnum"=w206) -> ()  [unwired: 2 in, 2 out]
            n134 = property on="Cal Value 4" class="DigNum (strict)"("DisabledEnum"=w206) -> ()  [unwired: 2 in, 2 out]
            n135 = property on="Cal Value 5" class="DigNum (strict)"("DisabledEnum"=w206) -> ()  [unwired: 2 in, 2 out]
            n136 = property on="1st Point Cal" class="Bool (strict)"("DisabledEnum"=w206) -> ()  [unwired: 2 in, 2 out]
            n137 = property on="2nd Point Cal" class="Bool (strict)"("DisabledEnum"=w206) -> ()  [unwired: 2 in, 2 out]
            n138 = property on="3rd Point Cal" class="Bool (strict)"("DisabledEnum"=w206) -> ()  [unwired: 2 in, 2 out]
            n139 = property on="5th Point Cal" class="Bool (strict)"("DisabledEnum"=w206) -> ()  [unwired: 2 in, 2 out]
            n140 = Select(t=string[] ["Calibrating 4"], s="4th Point Cal", f=string[] ["Stop Calibrating"]) -> (s? t:f=w207:string[])
          }
          event "5th Point Cal": Value Change {
            n141 = event-data() -> ()  [unwired: 1 in, 6 out]
            n142 = Select(t=T10."Disabled" ("Disabled"), s="5th Point Cal", f=T10."Enabled" ("Disabled")) -> (s? t:f=w214:T10)
            n143 = property on="Cal Value 1" class="DigNum (strict)"("DisabledEnum"=w214) -> ()  [unwired: 2 in, 2 out]
            n144 = property on="Cal Value 2" class="DigNum (strict)"("DisabledEnum"=w214) -> ()  [unwired: 2 in, 2 out]
            n145 = property on="Cal Value 3" class="DigNum (strict)"("DisabledEnum"=w214) -> ()  [unwired: 2 in, 2 out]
            n146 = property on="Cal Value 4" class="DigNum (strict)"("DisabledEnum"=w214) -> ()  [unwired: 2 in, 2 out]
            n147 = property on="Cal Value 5" class="DigNum (strict)"("DisabledEnum"=w214) -> ()  [unwired: 2 in, 2 out]
            n148 = property on="1st Point Cal" class="Bool (strict)"("DisabledEnum"=w214) -> ()  [unwired: 2 in, 2 out]
            n149 = property on="2nd Point Cal" class="Bool (strict)"("DisabledEnum"=w214) -> ()  [unwired: 2 in, 2 out]
            n150 = property on="3rd Point Cal" class="Bool (strict)"("DisabledEnum"=w214) -> ()  [unwired: 2 in, 2 out]
            n151 = property on="4th Point Cal" class="Bool (strict)"("DisabledEnum"=w214) -> ()  [unwired: 2 in, 2 out]
            n152 = Select(t=string[] ["Calibrating 5"], s="5th Point Cal", f=string[] ["Stop Calibrating"]) -> (s? t:f=w215:string[])
          }
          event "Cancel Verify": Value Change {
            n153 = event-data() -> ()  [unwired: 1 in, 1 out]
            n154 = Unbundle By Name(w221) -> ("StreamCtrlActive"=w219:bool, "Desired System.ID"=w220:string)
            n155 = case shown="True" w219 {
              tunnel: w220 -> [_ w223]
              frame False {
              }
              frame True {
                w224 = FALSE
                n156 = Format Into String(format string="ni.var.psp://10.30.189.%s/Streaming Control/StreamCalibrated", w223) -> (resulting string=w230:string, error out=w231:errorcluster)  [unwired: 2 in]
                n157 = shared-variable-open(w230, w231, w224) -> (w225:refnum<k21>, w228:errorcluster)  [unwired: 1 in]
                n158 = shared-variable-write(w225, w228, w224) -> (w226:refnum<k21>, w227:errorcluster)
                n159 = Close Variable Connection(8:w227, 11:w226) -> ()  [unwired: 1 out]
              }
            }
          }
          event "Verify Read": Value Change {
            n160 = event-data() -> ()  [unwired: 1 in, 1 out]
            n161 = case shown="False" "Verify Read" {
              tunnel: [FALSE ("Verify Read") FALSE ("Verify Read")] -> w238
              tunnel: w237 -> [_ _]
              tunnel: w237 -> [w242 w248]
              tunnel: [w242 w247] -> w236
              tunnel: [w240 string[] ["Calc Dev", "Cal Review"]] -> w233
              tunnel: w232 -> [w240 _]
              frame False {
              }
              frame True {
                n162 = local read "Ver Reading"() -> (w243:dbl)
                n163 = local read "Verify Table"() -> (w244:string[][])
                n164 = local read "Row"() -> (w251:i32)
                n165 = Number To Fractional String(number=w243) -> (F-format string=w250:string)  [unwired: 3 in]
                n166 = Replace Array Subset(array=w244, new element=w250, index (row)=w251, index (col)=1 ("disabled index (col)")) -> (w246:string[][])
                n167 = Increment(x=w251) -> (x+1=w255:i32)
                n168 = Bundle(w255, "disabled index (col)"=1) -> (w252:cluster{i32, "disabled index (col)":i32})  [unwired: 1 in]
                n169 = Bundle By Name(cluster=w248, "Verify Table"=w246) -> (w247:T9)
                n170 = property on="Verify Table" class="Tbl (strict)"("Key Focus"=TRUE, "EditPos"=w252, "Value"=w246) -> ()  [unwired: 2 in, 2 out]
              }
            }
            n171 = local write "Verify Read"(w238) -> ()
            n172 = Bundle By Name(cluster=w236, "Init Mean"=TRUE ("initialize")) -> (w235:T9)
          }
          event "Verify Edit": Value Change {
            n173 = event-data() -> ()  [unwired: 1 in, 1 out]
            n174 = case shown="False" "Verify Edit" {
              tunnel: w259 -> [w272 _]
              frame False {
                w273 = T10."Enabled" ("Disabled")
                n175 = Unbundle By Name(w272) -> ("Targets"=w268:T6, "Cal Targets Path"=w270:path, "Cal Unit"=w269:T2)
                n176 = local read "Verify Table"() -> (w271:string[][])
                n177 = Index Array(array=w271, index (col)=0 ("disabled index (col)")) -> (element=w262:string[])  [unwired: 1 in]
                n178 = Fract/Exp String To Number(string=w262) -> (number=w261:dbl[])  [unwired: 3 in, 1 out]
                n179 = Array To Cluster(array=w261) -> (cluster=w260:T14)
                n180 = case shown="\"A\"" w269 {
                  tunnel: w268 -> [w278 w281 w284 w287 w290]
                  tunnel: [w277 w280 w283 w286 w289] -> w267
                  tunnel: w260 -> [w276 w279 w282 w285 w288]
                  frame "V", Default {
                    n181 = Bundle By Name(cluster=w278, "V Targets"=w276) -> (w277:T6)
                  }
                  frame "mA" {
                    n182 = Bundle By Name(cluster=w281, "mA Targets"=w279) -> (w280:T6)
                  }
                  frame "A" {
                    n183 = Bundle By Name(cluster=w284, "A Targets"=w282) -> (w283:T6)
                  }
                  frame "Hz" {
                    n184 = Bundle By Name(cluster=w287, "Hz Targets"=w285) -> (w286:T6)
                  }
                  frame "deg C" {
                    n185 = Bundle By Name(cluster=w290, "TC Targets"=w288) -> (w289:T6)
                  }
                }
                n186 = call <vilib>:"Open Config Data.vi"("configuration file path"=w270) -> ("error out"=w266:errorcluster, "refnum"=w265:T15)  [unwired: 8 in, 1 out]
                n187 = call <userlib>:"Write INI Cluster__ogtk.vi"("error in (no error)"=w266, "INI Fomatted Cluster"=w267, "refnum"=w265) -> ("error out"=w264:errorcluster, "dup refnum"=w263:T15)  [unwired: 7 in]
                n188 = property on="Hide Cal Values" class="Bool"("Visible"=TRUE) -> ()  [unwired: 2 in, 2 out]
                n189 = call <vilib>:"Close Config Data.vi"("error in (no error)"=w264, "refnum"=w263) -> ()  [unwired: 8 in, 2 out]
                n190 = property on="Verify Read" class="Bool (strict)"("DisabledEnum"=w273) -> ()  [unwired: 2 in, 2 out]
                n191 = property on="Auto" class="Bool (strict)"("DisabledEnum"=w273) -> ()  [unwired: 2 in, 2 out]
              }
              frame True {
                w291 = T10."Disabled and Grayed Out" ("Disabled")
                n192 = property on="Verify Read" class="Bool (strict)"("DisabledEnum"=w291) -> ()  [unwired: 2 in, 2 out]
                n193 = property on="Auto" class="Bool (strict)"("DisabledEnum"=w291) -> ()  [unwired: 2 in, 2 out]
                n194 = property on="Hide Cal Values" class="Bool"("Visible"=FALSE) -> ()  [unwired: 2 in, 2 out]
              }
            }
          }
          event "Save Cal": Value Change {
            n195 = event-data() -> ()  [unwired: 1 in, 1 out]
            n196 = property on="Cal Table" class="Tbl (strict)"("DisabledEnum"=T10."Enabled" ("Disabled")) -> ()  [unwired: 2 in, 2 out]
            n197 = property on="Verify Tab" class="TabCtl (strict)"("Visible"=FALSE) -> ()  [unwired: 2 in, 2 out]
          }
          event "Auto": Value Change {
            n198 = event-data() -> ()  [unwired: 1 in, 1 out]
            n199 = case shown="True" "Auto" {
              frame False {
              }
              frame True {
                n200 = local read "Row"() -> (w301:i32)
                n201 = Bundle("Row"=w301, "disabled index (col)"=1) -> (w302:cluster{"Row":i32, "disabled index (col)":i32})  [unwired: 1 in]
                n202 = property on="Verify Table" class="Tbl (strict)"("Key Focus"=TRUE, "EditPos"=w302) -> ()  [unwired: 2 in, 2 out]
              }
            }
            n203 = Bundle By Name(cluster=w299, "Auto"="Auto") -> (w298:T9)
          }
          event "Verify Table": Value Change {
            n204 = event-data() -> ()  [unwired: 1 in, 1 out]
            n205 = Bundle By Name(cluster=w308, "Verify Table"="Verify Table") -> (w307:T9)
          }
          event "Confirm Cal Point": Value Change {
            w313 = T10."Enabled" ("Disabled")
            n206 = event-data() -> ()  [unwired: 1 in, 1 out]
            n207 = local read "Cal Reading"() -> (w317:dbl)
            n208 = Unbundle By Name(w320) -> ("LastCalPt"=w318:i32)
            n209 = flat-sequence {
              tunnel: w318 -> [w324]
              tunnel: w317 -> [w323]
              tunnel: FALSE -> [w322]
              tunnel: "Master Value" -> [w321]
              tunnel: [w340] -> w312
              frame #0 {
                n210 = case shown="0, Default" w324 {
                  tunnel: w323 -> [_ w325 w328 w331 w334 w337]
                  tunnel: w321 -> [_ w327 w330 w333 w336 w339]
                  tunnel: w322 -> [_ w326 w329 w332 w335 w338]
                  frame 0, Default {
                  }
                  frame 1 {
                    n211 = local write "Cal Value 1"(w327) -> ()
                    n212 = local write "1st Point Cal"(w326) -> ()
                    "Reading Value 1" <- w325
                  }
                  frame 2 {
                    n213 = local write "Cal Value 2"(w330) -> ()
                    n214 = local write "2nd Point Cal"(w329) -> ()
                    "Reading Value 2" <- w328
                  }
                  frame 3 {
                    n215 = local write "Cal Value 3"(w333) -> ()
                    n216 = local write "3rd Point Cal"(w332) -> ()
                    "Reading Value 3" <- w331
                  }
                  frame 4 {
                    n217 = local write "Cal Value 4"(w336) -> ()
                    n218 = local write "4th Point Cal"(w335) -> ()
                    "Reading Value 4" <- w334
                  }
                  frame 5 {
                    n219 = local write "Cal Value 5"(w339) -> ()
                    n220 = local write "5th Point Cal"(w338) -> ()
                    "Reading Value 5" <- w337
                  }
                }
              }
              frame #1 {
                n221 = local read "Reading Value 2"() -> (w345:dbl)
                n222 = local read "Reading Value 3"() -> (w346:dbl)
                n223 = local read "Reading Value 4"() -> (w347:dbl)
                n224 = local read "Reading Value 5"() -> (w348:dbl)
                n225 = Not Equal To 0?(x=w345) -> (x != 0?=w344:bool)
                n226 = Not Equal To 0?(x=w346) -> (x != 0?=w343:bool)
                n227 = Not Equal To 0?(x=w347) -> (x != 0?=w342:bool)
                n228 = Not Equal To 0?(x=w348) -> (x != 0?=w341:bool)
                n229 = Compound Arithmetic op=AND(w344, w343, w342, w341) -> (w340:bool)
              }
            }
            n230 = property on="Cal Value 1" class="DigNum (strict)"("DisabledEnum"=w313) -> ()  [unwired: 2 in, 2 out]
            n231 = property on="Cal Value 2" class="DigNum (strict)"("DisabledEnum"=w313) -> ()  [unwired: 2 in, 2 out]
            n232 = property on="Cal Value 3" class="DigNum (strict)"("DisabledEnum"=w313) -> ()  [unwired: 2 in, 2 out]
            n233 = property on="Cal Value 4" class="DigNum (strict)"("DisabledEnum"=w313) -> ()  [unwired: 2 in, 2 out]
            n234 = property on="Cal Value 5" class="DigNum (strict)"("DisabledEnum"=w313) -> ()  [unwired: 2 in, 2 out]
            n235 = property on="1st Point Cal" class="Bool (strict)"("DisabledEnum"=w313) -> ()  [unwired: 2 in, 2 out]
            n236 = property on="2nd Point Cal" class="Bool (strict)"("DisabledEnum"=w313) -> ()  [unwired: 2 in, 2 out]
            n237 = property on="3rd Point Cal" class="Bool (strict)"("DisabledEnum"=w313) -> ()  [unwired: 2 in, 2 out]
            n238 = property on="4th Point Cal" class="Bool (strict)"("DisabledEnum"=w313) -> ()  [unwired: 2 in, 2 out]
            n239 = property on="5th Point Cal" class="Bool (strict)"("DisabledEnum"=w313) -> ()  [unwired: 2 in, 2 out]
            n240 = local write "Cal Tab"(enum32{"Apply", "Cal"}."Apply" ("Cal Tab")) -> ()
            n241 = Select(t=T10."Enabled" ("Disabled"), s=w312, f=T10."Disabled and Grayed Out" ("Disabled")) -> (s? t:f=w309:T10)
            n242 = property on="Apply Cal" class="Bool"("DisabledEnum"=w309) -> ()  [unwired: 2 in, 2 out]
          }
          event "Apply Cal": Value Change {
            n243 = event-data() -> ()  [unwired: 1 in, 6 out]
            n244 = Insert Into Array(array=w352, index=0, new element=string[] ["Calculate Coeffs"]) -> (w351:string[])
          }
          event "Start Verification": Value Change {
            n245 = event-data() -> ()  [unwired: 1 in, 6 out]
            n246 = Unbundle By Name(w356) -> ("StreamCtrlActive"=w354:bool, "Desired System.ID"=w355:string)
            n247 = case shown="True" w354 {
              tunnel: w355 -> [_ w362]
              frame False {
              }
              frame True {
                n248 = Format Into String(format string="ni.var.psp://10.30.189.%s/Streaming Control/StreamCalibrated", w362) -> (resulting string=w370:string, error out=w371:errorcluster)  [unwired: 2 in]
                n249 = shared-variable-open(w370, w371, FALSE) -> (w364:refnum<k21>, w367:errorcluster)  [unwired: 1 in]
                n250 = shared-variable-write(w364, w367, TRUE ("data in")) -> (w365:refnum<k21>, w366:errorcluster)
                n251 = Close Variable Connection(8:w366, 11:w365) -> ()  [unwired: 1 out]
              }
            }
            n252 = property on="Verify Tab" class="TabCtl (strict)"("Visible"="Start Verification") -> ()  [unwired: 2 in, 2 out]
            n253 = Insert Into Array(array=w358, index=0, new element=string[] ["Load Targets", "Calculate Coeffs"]) -> (w357:string[])
          }
          event "Cancel Cal": Value Change {
            w383 = T10."Disabled and Grayed Out" ("Disabled")
            w379 = T10."Enabled" ("Disabled")
            n254 = event-data() -> ()  [unwired: 1 in, 6 out]
            n255 = Unbundle By Name(w375) -> ("Desired System.ID"=w378:string)
            n256 = Format Into String(format string="10.30.189.%s", w378) -> (resulting string=w374:string)  [unwired: 2 in, 1 out]
            n257 = property on="Header" class="Bool"("DisabledEnum"=w379) -> ()  [unwired: 2 in, 2 out]
            n258 = property on="Channel to Cal" class="Enum (strict)"("DisabledEnum"=w379) -> ()  [unwired: 2 in, 2 out]
            n259 = property on="View Spreadsheet" class="Bool"("DisabledEnum"=w379) -> ()  [unwired: 2 in, 2 out]
            n260 = flat-sequence {
              tunnel: w374 -> [w385]
              tunnel: [w385] -> w372
              tunnel: [w388] -> w373
              tunnel: w372 -> [w388]
              frame #0 {
                n261 = local write "RIO Found"(FALSE ("RIO Found")) -> ()
              }
              frame #1 {
                n262 = Wait (ms)(milliseconds to wait=u32 20) -> ()  [unwired: 1 out]
              }
            }
            n263 = property on="Start Cal" class="Bool"("DisabledEnum"=w379) -> ()  [unwired: 2 in, 2 out]
            n264 = disable-structure shown="Disabled" {
              disable-tunnel: w379 -> [w384 _]
              frame Disabled {
                n265 = property on="Start Verification" class="Bool"("DisabledEnum"=w384) -> ()  [unwired: 2 in, 2 out]
              }
              frame Enabled {
              }
            }
            n266 = call "TCP Data Stream PC.vi"("RT IP Address"=w373, "Mode"=TCP_Data_Stream_Mode_(PC)."Close") -> ()  [unwired: 14 in, 4 out]
            n267 = property on="Cal Tab" class="TabCtl (strict)"("Visible"=FALSE) -> ()  [unwired: 2 in, 2 out]
            n268 = property on="Cal Unit" class="Enum (strict)"("DisabledEnum"=T10."Enabled" ("Disabled")) -> ()  [unwired: 2 in, 2 out]
            n269 = property on="Reading Value 1" class="DigNum (strict)"("DisabledEnum"=w383) -> ()  [unwired: 2 in, 2 out]
            n270 = property on="Cal Value 1" class="DigNum (strict)"("DisabledEnum"=w383) -> ()  [unwired: 2 in, 2 out]
            n271 = property on="1st Point Cal" class="Bool (strict)"("DisabledEnum"=w383) -> ()  [unwired: 2 in, 2 out]
            n272 = property on="Reading Value 2" class="DigNum (strict)"("DisabledEnum"=w383) -> ()  [unwired: 2 in, 2 out]
            n273 = property on="Cal Value 2" class="DigNum (strict)"("DisabledEnum"=w383) -> ()  [unwired: 2 in, 2 out]
            n274 = property on="2nd Point Cal" class="Bool (strict)"("DisabledEnum"=w383) -> ()  [unwired: 2 in, 2 out]
            n275 = property on="Reading Value 3" class="DigNum (strict)"("DisabledEnum"=w383) -> ()  [unwired: 2 in, 2 out]
            n276 = property on="Cal Value 3" class="DigNum (strict)"("DisabledEnum"=w383) -> ()  [unwired: 2 in, 2 out]
            n277 = property on="3rd Point Cal" class="Bool (strict)"("DisabledEnum"=w383) -> ()  [unwired: 2 in, 2 out]
            n278 = property on="Reading Value 4" class="DigNum (strict)"("DisabledEnum"=w383) -> ()  [unwired: 2 in, 2 out]
            n279 = property on="Cal Value 4" class="DigNum (strict)"("DisabledEnum"=w383) -> ()  [unwired: 2 in, 2 out]
            n280 = property on="4th Point Cal" class="Bool (strict)"("DisabledEnum"=w383) -> ()  [unwired: 2 in, 2 out]
            n281 = property on="Reading Value 5" class="DigNum (strict)"("DisabledEnum"=w383) -> ()  [unwired: 2 in, 2 out]
            n282 = property on="Cal Value 5" class="DigNum (strict)"("DisabledEnum"=w383) -> ()  [unwired: 2 in, 2 out]
            n283 = property on="5th Point Cal" class="Bool (strict)"("DisabledEnum"=w383) -> ()  [unwired: 2 in, 2 out]
          }
          event "Transfer Cal": Value Change {
            n284 = event-data() -> ()  [unwired: 1 in, 6 out]
            n285 = disable-structure shown="Enabled" {
              disable-tunnel: [string[] ["Distribute Calibration"] w393] -> w390
              disable-tunnel: w389 -> [_ w393]
              frame Disabled {
              }
              frame Enabled {
              }
            }
          }
          event Value Change {
            n286 = event-data() -> ()  [unwired: 1 in, 1 out]
            n287 = Bundle By Name(cluster=w397, "Cal Unit"="Cal Unit") -> (w396:T9)
          }
        }
      }
      frame "Init" {
        w404 = FALSE ("Visible")
        w409 = Units_Type_Def_(DAQ_Rack)."A" ("Cal Unit")
        # "#Change adding in\nnew subVI for RIO"
        n288 = Unbundle By Name(w418) -> ("debug"=w417:bool, "App Dir"=w416:path)
        n289 = Select(t=path "C:/Users/zstreeter/Documents/Projects/Calibration Utility/Source", s=w417, f=w416) -> (s? t:f=w415:path)
        n290 = Build Path(base path=w415, name or relative path="App Config.ini") -> (appended path=w421:path)
        n291 = Build Path(base path=w415, name or relative path="Calibration UIs\\Gas Rack") -> (appended path=w413:path)
        n292 = call "Read App Config.vi"("App Config Path"=w421) -> ("Cal Files Path"=w424:path, "Registered Systems"=w411:T3[])  [unwired: 9 in]
        n293 = Build Path(base path=w424, name or relative path="Gas Rack") -> (appended path=w420:path)
        n294 = Build Path(base path=w413, name or relative path="Gas Rack Cal Targets.ini") -> (appended path=w423:path)
        n295 = Create Folder(path (use dialog)=w420) -> (error out=w426:errorcluster)  [unwired: 2 in, 2 out]
        n296 = call <vilib>:"Clear Errors.vi"("error in (no error)"=w426) -> ("error out"=w419:errorcluster)  [unwired: 5 in, 1 out]
        n297 = for {
          tunnel: [w434] -> w412 mode=indexing
          tunnel: w420 -> [w433]
          tunnel: w419 -> [w432]
          tunnel: w413 -> [w431]
          tunnel: string[] ["Gas Rack Cal Template.xls"] -> [w430] mode=indexing
          n298 = Build Path(base path=w433, name or relative path=w430) -> (appended path=w434:path)
          n299 = Build Path(base path=w431, name or relative path=w430) -> (appended path=w437:path)
          n300 = call <vilib>:"Check if File or Folder Exists.vi"("error in (no error)"=w432, "path"=w434) -> ("file or folder exists?"=w435:bool, "dup path"=w436:path)  [unwired: 7 in, 1 out]
          n301 = case shown="True" w435 {
            tunnel: w436 -> [w439 _]
            tunnel: w437 -> [w438 _]
            frame False {
              n302 = Copy(10:w439, 11:w438) -> ()  [unwired: 3 in, 3 out]
            }
            frame True {
            }
          }
        }
        n303 = Index Array(array=w412) -> (element=w408:path)  [unwired: 1 in]
        n304 = call "Gas Rack Create Cal File Array (RIO).vi"() -> ("Cal Target Array"=w398:string[], "Cal Log OUT"=w399:string[][])  [unwired: 10 in]
        n305 = Bundle By Name(cluster=w418, "Registered Systems"=w411, "Cal Files Base Path"=w420, "Base Path"=w415, "Cal Targets Path"=w423, "Cal Template Path"=w408, "Default Cal Log"=w399, "Cal Target Array"=w398, "Cal Unit"=w409) -> (w403:T9)
        n306 = property on="Cal Tab" class="TabCtl (strict)"("Visible"=w404) -> ()  [unwired: 2 in, 2 out]
        n307 = property on="Verify Tab" class="TabCtl (strict)"("Visible"=w404) -> ()  [unwired: 2 in, 2 out]
        n308 = local write "Tank IP:"("" ("DAQ Rack")) -> ()
        n309 = local write "Cal Table"(string[][] []) -> ()
        n310 = local write "Cal Unit"(w409) -> ()
        n311 = flat-sequence {
          tunnel: w403 -> [w429]
          tunnel: [w429] -> w402
          tunnel: w401 -> [w428]
          frame #0 {
            n312 = Set Occurrence(w428) -> ()
          }
        }
      }
      frame "Unused Items" {
      }
      frame "Init Cal" {
        w444 = FALSE ("Auto")
        w450 = FALSE ("Verify Read")
        w451 = T10."Enabled" ("Disabled")
        w443 = FALSE ("Visible")
        w442 = T10."Disabled and Grayed Out" ("Disabled")
        n313 = Unbundle By Name(w454) -> ("Cal Log Header"=w446:string[])
        n314 = property on="Cal Table" class="Tbl (strict)"("Column Headers[]"=w446) -> ()  [unwired: 2 in, 2 out]
        n315 = property on="Reading Value 1" class="DigNum (strict)"("DisabledEnum"=w442) -> ()  [unwired: 2 in, 2 out]
        n316 = property on="Cal Value 1" class="DigNum (strict)"("DisabledEnum"=w442) -> ()  [unwired: 2 in, 2 out]
        n317 = property on="1st Point Cal" class="Bool (strict)"("DisabledEnum"=w442) -> ()  [unwired: 2 in, 2 out]
        n318 = property on="Reading Value 2" class="DigNum (strict)"("DisabledEnum"=w442) -> ()  [unwired: 2 in, 2 out]
        n319 = property on="Cal Value 2" class="DigNum (strict)"("DisabledEnum"=w442) -> ()  [unwired: 2 in, 2 out]
        n320 = property on="2nd Point Cal" class="Bool (strict)"("DisabledEnum"=w442) -> ()  [unwired: 2 in, 2 out]
        n321 = property on="Reading Value 3" class="DigNum (strict)"("DisabledEnum"=w442) -> ()  [unwired: 2 in, 2 out]
        n322 = property on="Cal Value 3" class="DigNum (strict)"("DisabledEnum"=w442) -> ()  [unwired: 2 in, 2 out]
        n323 = property on="3rd Point Cal" class="Bool (strict)"("DisabledEnum"=w442) -> ()  [unwired: 2 in, 2 out]
        n324 = property on="Reading Value 4" class="DigNum (strict)"("DisabledEnum"=w442) -> ()  [unwired: 2 in, 2 out]
        n325 = property on="Cal Value 4" class="DigNum (strict)"("DisabledEnum"=w442) -> ()  [unwired: 2 in, 2 out]
        n326 = property on="4th Point Cal" class="Bool (strict)"("DisabledEnum"=w442) -> ()  [unwired: 2 in, 2 out]
        n327 = property on="Reading Value 5" class="DigNum (strict)"("DisabledEnum"=w442) -> ()  [unwired: 2 in, 2 out]
        n328 = property on="Cal Value 5" class="DigNum (strict)"("DisabledEnum"=w442) -> ()  [unwired: 2 in, 2 out]
        n329 = property on="5th Point Cal" class="Bool (strict)"("DisabledEnum"=w442) -> ()  [unwired: 2 in, 2 out]
        n330 = property on="Verify Read" class="Bool (strict)"("DisabledEnum"=w451) -> ()  [unwired: 2 in, 2 out]
        n331 = property on="Cal Table" class="Tbl (strict)"("DisabledEnum"=w451) -> ()  [unwired: 2 in, 2 out]
        n332 = property on="Verify Tab" class="TabCtl (strict)"("Visible"=w443) -> ()  [unwired: 2 in, 2 out]
        n333 = property on="Cal Tab" class="TabCtl (strict)"("Visible"=w443) -> ()  [unwired: 2 in, 2 out]
        n334 = property on="Hide Cal Values" class="Bool"("Visible"=TRUE) -> ()  [unwired: 2 in, 2 out]
        n335 = local write "Verify Read"(w450) -> ()
        n336 = local write "Auto"(w450) -> ()
        n337 = local write "Verify Edit"(w450) -> ()
        n338 = Bundle By Name(cluster=w454, "Auto"=w444, "Verification"=w444) -> (w453:T9)
        n339 = Insert Into Array(array=w448, index=0, new element=string[] ["Clear Dev Data", "Update Dev Tables", "Load Template"]) -> (w445:string[])
      }
      frame "Check for RIO" {
        n340 = Unbundle By Name(w462) -> ("Desired System.Serial Number"=w457:u32, "StreamCtrlActive"=w455:bool, "Desired System.ID"=w459:string, "Verification"=w460:bool)
        n341 = local read "RIO Found"() -> (w458:bool)
        n342 = local write "Lost Connection"(FALSE ("Lost Connection")) -> ()
        n343 = case shown="False" w458 {
          selector: w458 -> [w468 _]
          tunnel: [string[] [] w476] -> w463
          tunnel: [w468 w475] -> w461
          tunnel: w460 -> [_ w474]
          tunnel: w455 -> [_ w473]
          tunnel: w459 -> [_ w472]
          tunnel: w457 -> [_ w469]
          frame True {
          }
          frame False {
            n344 = call "Find Network Systems.vi"() -> ("Serial Number"=w471:u32)  [unwired: 10 in, 1 out]
            n345 = Equal?(x=w471, y=w469) -> (x = y?=w470:bool)
            n346 = case shown="True" w470 {
              selector: w470 -> [w479 w495]
              tunnel: w474 -> [w480 _]
              tunnel: [w481 string[] []] -> w476
              tunnel: [w479 w495] -> w475
              tunnel: w472 -> [w478 _]
              tunnel: w473 -> [w477 _]
              frame True {
                # "Desired system found."
                n347 = case shown="True" w477 {
                  tunnel: w478 -> [_ w482]
                  frame False {
                  }
                  frame True {
                    w483 = FALSE
                    n348 = Format Into String(format string="ni.var.psp://10.30.189.%s/Streaming Control/StreamCalibrated", w482) -> (resulting string=w489:string, error out=w490:errorcluster)  [unwired: 2 in]
                    n349 = shared-variable-open(w489, w490, w483) -> (w484:refnum<k21>, w487:errorcluster)  [unwired: 1 in]
                    n350 = shared-variable-write(w484, w487, w483) -> (w485:refnum<k21>, w486:errorcluster)
                    n351 = Close Variable Connection(8:w486, 11:w485) -> ()  [unwired: 1 out]
                  }
                }
                n352 = case shown="True" w480 {
                  tunnel: [string[] ["Load Targets", "Calculate Coeffs"] w492] -> w481
                  frame True {
                  }
                  frame False {
                    n353 = disable-structure shown="Enabled" {
                      disable-tunnel: [string[] ["Load Targets", "Start Cal"] string[] ["Load Targets"]] -> w492
                      frame Disabled {
                      }
                      frame Enabled {
                      }
                    }
                  }
                }
              }
              frame False {
                # "Couldn't find desired system."
                n354 = property on="Header" class="Bool"("DisabledEnum"=T10."Enabled" ("Disabled")) -> ()  [unwired: 2 in, 2 out]
                n355 = One Button Dialog(message="Couldn't connect to desired DAQ hardware.") -> ()  [unwired: 1 in, 1 out]
              }
            }
          }
        }
        "RIO Found" <- w461
        n356 = Insert Into Array(array=w465, index=0, new element=w463) -> (w464:string[])
      }
      frame "Adjust Channels" {
        n357 = Unbundle By Name(w513) -> ("Cal Unit"=w507:T2)
        n358 = property on="Channel to Cal" class="Enum (strict)"() -> ("NumItems"=w500:u32)  [unwired: 2 in, 2 out]
        n359 = property on="Cal Unit" class="Enum (strict)"() -> ("Strings []"=w510:string[])  [unwired: 2 in, 2 out]
        n360 = for {
          N: w500 -> [_]
          shift-right: [w527] -> w503
          shift-left: i32[] [] ("Disabled Items []") -> [w528]
          i -> [w526]
          n361 = case shown="7" w526 {
            tunnel: w528 -> [w529 w532]
            tunnel: [w529 w530] -> w527
            tunnel: w526 -> [_ w531]
            frame 0..6, Default {
            }
            frame 7 {
              n362 = Build Array (concatenate)(w532, w531) -> (w530:i32[])
            }
          }
        }
        n363 = for {
          tunnel: w510 -> [w521] mode=indexing
          shift-right: [w519] -> w502
          shift-left: i32[] [] ("Disabled Items []") -> [w520]
          i -> [w518]
          n364 = case shown="\"Hz\", \"deg C\", \"mA\"" w521 {
            tunnel: w520 -> [w522 w525]
            tunnel: [w522 w523] -> w519
            tunnel: w518 -> [_ w524]
            frame "A", "V", Default {
            }
            frame "Hz", "deg C", "mA" {
              n365 = Build Array (concatenate)(w525, w524) -> (w523:i32[])
            }
          }
        }
        n366 = Search 1D Array(1D array=w502, element=w507) -> (index of element=w509:i32)  [unwired: 1 in]
        n367 = disable-structure shown="Enabled" {
          disable-tunnel: w503 -> [w516 _]
          disable-tunnel: w502 -> [w515 _]
          disable-tunnel: [w516 w517] -> w499
          disable-tunnel: [w515 w517] -> w501
          frame Disabled {
          }
          frame Enabled {
            w517 = i32[] [] ("Disabled Items []")
          }
        }
        n368 = Greater Or Equal To 0?(x=w509) -> (x >= 0?=w508:bool)
        n369 = case shown="True" w508 {
          tunnel: [w533 w534] -> w506
          tunnel: w507 -> [w533 _]
          tunnel: w502 -> [_ w536]
          frame False {
          }
          frame True {
            n370 = for {
              N: 5 -> [_]
              tunnel: w536 -> [w540]
              tunnel: [w537] -> w534
              i -> [w537]
              stop <- w538 stop-if-true
              n371 = Search 1D Array(1D array=w540, element=w537) -> (index of element=w539:i32)  [unwired: 1 in]
              n372 = Less Than 0?(x=w539) -> (x < 0?=w538:bool)
            }
            n373 = local write "Cal Unit"(w534) -> ()
          }
        }
        n374 = property on="Channel to Cal" class="Enum (strict)"("Disabled Items []"=w499) -> ()  [unwired: 2 in, 2 out]
        n375 = property on="Cal Unit" class="Enum (strict)"("Disabled Items []"=w501) -> ()  [unwired: 2 in, 2 out]
        n376 = Bundle By Name(cluster=w513, "Rack Version"=Rack_Version_Type_Def."RIO", "Cal Unit"=w506) -> (w512:T9)
      }
      frame "Clear Dev Data" {
        n377 = Bundle By Name(cluster=w543, "Verify Table"=string[][] [["", "", "", "", ""], ["", "", "", "", ""], ["", "", "", "", ""], ["", "", "", "", ""], ["", "", "", "", ""], ["", "", "", "", ""], ["", "", "", "", ""], ["", "", "", "", ""], ["", "", "", "", ""], ["", "", "", "", ""]]) -> (w542:T9)
      }
      frame "Update Dev Tables" {
        n378 = Unbundle By Name(w546) -> ("Verify Table"=w545:string[][])
        n379 = local write "Verify Table"(w545) -> ()
      }
      frame "Load Template" {
        n380 = Unbundle By Name(w549) -> ("Cal Template Path"=w554:path)
        n381 = call <vilib>:"Check if File or Folder Exists.vi"("path"=w554) -> ("file or folder exists?"=w553:bool)  [unwired: 8 in, 2 out]
        n382 = case shown="False" w553 {
          tunnel: [string[] [] string[] []] -> w552
          tunnel: w554 -> [w561 w564]
          tunnel: [FALSE ("Visible") FALSE ("Visible")] -> w555
          tunnel: [w558 w566] -> w556
          tunnel: [w558 w566] -> w557
          frame False {
            w558 = T10."Disabled and Grayed Out" ("Disabled")
            n383 = Format Into String(format string="Can't find cal spreadsheet template!\n\nShould have been here:  \"%s\"" ("message"), w561) -> (resulting string=w560:string)  [unwired: 2 in, 1 out]
            n384 = One Button Dialog(message=w560) -> ()  [unwired: 1 in, 1 out]
          }
          frame True {
            w566 = T10."Enabled" ("Disabled")
            n385 = call "Read Write Header.vi"("Cal Template Path"=w564, "Write (F)"=FALSE) -> ("Header Table 1"=w572:string[][], "Header Table 2"=w571:string[][], "Sys Cal Table"=w568:string[][], "Cal Standards Table"=w567:string[][], "Header Comments"=w569:string[][])  [unwired: 13 in]
            n386 = local write "Header Table 1"(w572) -> ()
            n387 = local write "Header Table 2"(w571) -> ()
            n388 = local write "Sys Cal Table"(w568) -> ()
            n389 = local write "Cal Standards Table"(w567) -> ()
            n390 = local write "Header Comments"(w569) -> ()
          }
        }
        n391 = property on="Load Indicator Tab" class="TabCtl (strict)"("Visible"=w555) -> ()  [unwired: 2 in, 2 out]
        n392 = property on="Header OK" class="Bool"("DisabledEnum"=w556) -> ()  [unwired: 2 in, 2 out]
        n393 = property on="Header Cancel" class="Bool"("DisabledEnum"=w557) -> ()  [unwired: 2 in, 2 out]
        n394 = Insert Into Array(array=w551, index=0, new element=w552) -> (w550:string[])
      }
      frame "Create Spreadsheet" {
        n395 = Unbundle By Name(w585) -> ("Rack Version"=w580:T5, "DAQ Rack"=w577:string, "Cal Files Base Path"=w587:path)
        n396 = Format Into String(format string="%s.xls", w577) -> (resulting string=w576:string)  [unwired: 2 in, 1 out]
        n397 = case shown="\"RIO\"" w580 {
          tunnel: ["DAQ Rack Cal Template.xls" ("name or relative path") "DAQ Cart Cal Template.xls" ("name or relative path") "Gas Rack Cal Template.xls" ("name or relative path")] -> w575
          frame Default {
          }
          frame "Cart" {
          }
          frame "RIO" {
          }
        }
        n398 = Build Path(base path=w587, name or relative path=w576) -> (appended path=w574:path)
        n399 = Empty String/Path?(string/path=w577) -> (empty?=w579:bool)
        n400 = Not A Number/Path/Refnum?(number/path/refnum=w574) -> (NaN/Path/Refnum?=w589:bool)
        n401 = Or(x=w589, y=w579) -> (x .or. y?=w590:bool)
        n402 = Build Path(base path=w587, name or relative path=w575) -> (appended path=w588:path)
        n403 = case shown="False" w590 {
          tunnel: [string[] ["Save Header"] string[] []] -> w586
          tunnel: w574 -> [w595 _]
          tunnel: w588 -> [w596 _]
          frame False {
            n404 = call <vilib>:"Check if File or Folder Exists.vi"("path"=w595) -> ("file or folder exists?"=w594:bool)  [unwired: 8 in, 2 out]
            n405 = case shown="False" w594 {
              tunnel: w595 -> [w600 _]
              tunnel: w596 -> [w599 _]
              frame False {
                n406 = Copy(9:TRUE ("overwrite (F)"), 10:w600, 11:w599) -> ()  [unwired: 2 in, 3 out]
              }
              frame True {
              }
            }
          }
          frame True {
            w601 = T10."Enabled" ("Disabled")
            n407 = property on="Load Indicator Tab" class="TabCtl (strict)"("Visible"=FALSE) -> ()  [unwired: 2 in, 2 out]
            n408 = property on="Header OK" class="Bool"("DisabledEnum"=w601) -> ()  [unwired: 2 in, 2 out]
            n409 = property on="Header Cancel" class="Bool"("DisabledEnum"=w601) -> ()  [unwired: 2 in, 2 out]
            n410 = One Button Dialog(message="\"Manufacturer Serial #\" is blank or contains invalid characters.") -> ()  [unwired: 1 in, 1 out]
          }
        }
        n411 = Bundle By Name(cluster=w585, "Cal Spreadsheet Path"=w574) -> (w584:T9)
        n412 = Insert Into Array(array=w582, index=0, new element=w586) -> (w583:string[])
      }
      frame "Save Header" {
        n413 = Unbundle By Name(w613) -> ("Cal Spreadsheet Path"=w616:path, "Cal Template Path"=w617:path)
        n414 = Build Array(w616, w617) -> (w618:path[])
        n415 = for {
          tunnel: "Header Table 2" -> [w626]
          tunnel: "Sys Cal Table" -> [w625]
          tunnel: "Cal Standards Table" -> [w624]
          tunnel: "Header Comments" -> [w623]
          tunnel: [w622] -> w615
          tunnel: "Header Table 1" -> [w620]
          tunnel: w618 -> [w619] mode=indexing
          n416 = call "Read Write Header.vi"("Header Table 1 IN"=w620, "Header Table 2 IN"=w626, "Sys Cal Table IN"=w625, "Cal Standards Table IN"=w624, "Header Comments IN"=w623, "Cal Template Path"=w619, "Write (F)"=TRUE) -> ("Header Table 1"=w622:string[][])  [unwired: 8 in, 4 out]
        }
        n417 = flat-sequence {
          tunnel: w615 -> [_]
          frame #0 {
            w627 = T10."Enabled" ("Disabled")
            w629 = FALSE ("Visible")
            n418 = disable-structure shown="Disabled" {
              disable-tunnel: w627 -> [w630 _]
              frame Disabled {
                n419 = property on="Start Verification" class="Bool"("DisabledEnum"=w630) -> ()  [unwired: 2 in, 2 out]
              }
              frame Enabled {
              }
            }
            n420 = property on="View Spreadsheet" class="Bool"("DisabledEnum"=w627) -> ()  [unwired: 2 in, 2 out]
            n421 = property on="Main Tab" class="TabCtl (strict)"("DisabledEnum"=w627) -> ()  [unwired: 2 in, 2 out]
            n422 = property on="Tank IP:" class="Str"("DisabledEnum"=w627) -> ()  [unwired: 2 in, 2 out]
            n423 = property on="Channel to Cal" class="Enum (strict)"("DisabledEnum"=w627) -> ()  [unwired: 2 in, 2 out]
            n424 = property on="Start Cal" class="Bool"("DisabledEnum"=w627) -> ()  [unwired: 2 in, 2 out]
            n425 = property on="Cal Unit" class="Enum (strict)"("DisabledEnum"=T10."Enabled" ("Disabled")) -> ()  [unwired: 2 in, 2 out]
            n426 = property on="Load Indicator Tab" class="TabCtl (strict)"("Visible"=w629) -> ()  [unwired: 2 in, 2 out]
            n427 = property on="Header Tab" class="TabCtl (strict)"("Visible"=w629) -> ()  [unwired: 2 in, 2 out]
          }
        }
        n428 = Insert Into Array(array=w611, index=0, new element=string[] []) -> (w612:string[])
      }
      frame "Create Cal File" {
        n429 = Unbundle By Name(w634) -> ("Cal Files Base Path"=w636:path, "Cal Log Header"=w639:string[], "Default Cal Log"=w638:string[][])
        n430 = local read "Tank IP:"() -> (w631:string)
        n431 = Build Array (concatenate)(w639, w638) -> (w637:string[][])
        n432 = case shown="Default" w631 {
          tunnel: w637 -> [w648 _]
          tunnel: w636 -> [w647 _]
          tunnel: w631 -> [w645 _]
          tunnel: [w646 path "" ("dup path")] -> w632
          frame Default {
            n433 = Format Into String(format string="%s.cal", w645) -> (resulting string=w643:string)  [unwired: 2 in, 1 out]
            n434 = Build Path(base path=w647, name or relative path=w643) -> (appended path=w651:path)
            n435 = call <vilib>:"Check if File or Folder Exists.vi"("path"=w651) -> ("file or folder exists?"=w650:bool, "dup path"=w649:path)  [unwired: 8 in, 1 out]
            n436 = case shown="False" w650 {
              tunnel: w649 -> [w655 w656]
              tunnel: w648 -> [w654 _]
              tunnel: [w652 w656] -> w646
              frame False {
                n437 = call-poly <vilib>:"Write To Spreadsheet File.vi"("delimiter (\\t)"="," ("delimiter (\\t)"), "2D data"=w654, "file path (dialog if empty)"=w655) -> ("new file path (Not A Path if cancelled)"=w652:path)  [unwired: 5 in]
              }
              frame True {
              }
            }
          }
          frame "" {
          }
        }
        n438 = Bundle By Name(cluster=w634, "Cal File Path"=w632) -> (w633:T9)
        n439 = Insert Into Array(array=w640, index=0, new element=string[] ["Load Cal File"]) -> (w641:string[])
      }
      frame "Load Cal File" {
        n440 = Unbundle By Name(w662) -> ("Default Cal Log"=w658:string[][], "Cal File Path"=w659:path)
        n441 = Empty String/Path?(string/path=w659) -> (empty?=w660:bool)
        n442 = case shown="False" w660 {
          tunnel: w659 -> [w669 _]
          tunnel: [w673 w710] -> w666
          tunnel: [w671 string[] []] -> w663
          tunnel: w662 -> [w670 w710]
          tunnel: w658 -> [w667 _]
          frame False {
            n443 = call <vilib>:"Check if File or Folder Exists.vi"("path"=w669) -> ("file or folder exists?"=w672:bool, "dup path"=w668:path)  [unwired: 8 in, 1 out]
            n444 = case shown="True" w672 {
              tunnel: w668 -> [_ w704]
              tunnel: w670 -> [w674 w701]
              tunnel: [w674 w700] -> w673
              tunnel: [string[] ["Create Cal File"] string[] []] -> w671
              tunnel: w667 -> [_ w697]
              frame False {
              }
              frame True {
                w696 = 0 ("index (row)")
                n445 = call-poly <vilib>:"Read From Spreadsheet File.vi"("delimiter (\\t)"="," ("delimiter (\\t)"), "file path (dialog if empty)"=w704) -> ("all rows"=w703:string[][])  [unwired: 5 in, 4 out]
                n446 = Delete From Array(array=w703, index (row)=0) -> (array with subset deleted=w692:string[][])  [unwired: 2 in, 1 out]
                n447 = Index Array(array=w692, index (col)=0 ("disabled index (col)")) -> (element=w694:string[])  [unwired: 1 in]
                n448 = Search 1D Array(1D array=w694, element="") -> (index of element=w690:i32)  [unwired: 1 in]
                n449 = Delete From Array(array=w692, index (row)=w690) -> (array with subset deleted=w691:string[][])  [unwired: 2 in, 1 out]
                n450 = Replace Array Subset(array=w697, new element=w691, index (row)=w696, index (col)=w696) -> (w684:string[][])
                n451 = Index Array(array=w684, index (col)=1 ("disabled index (col)")) -> (element=w677:string[])  [unwired: 1 in]
                n452 = for {
                  tunnel: w677 -> [w706] mode=indexing
                  tunnel: [w705] -> w676 mode=indexing
                  n453 = case shown="\"V\", Default" w706 {
                    tunnel: ["V" "A"] -> w705
                    frame "V", Default {
                    }
                    frame "A" {
                    }
                  }
                }
                n454 = Array To Spreadsheet String(array=w676, 3:"%s" ("format string")) -> (spreadsheet string=w688:string)  [unwired: 1 in]
                n455 = Search and Replace String(replace all?=TRUE ("replace all? (F)"), input string=w688, search string="degC", replace string="deg C" ("search string")) -> (result string=w681:string)  [unwired: 4 in, 3 out]
                n456 = Spreadsheet String To Array(format string="%s", spreadsheet string=w681, array type (2D Dbl)=w676) -> (array=w680:string[])  [unwired: 1 in]
                n457 = Replace Array Subset(array=w684, new element=w680, index (col)=1 ("disabled index (col)")) -> (w683:string[][])  [unwired: 1 in]
                n458 = Bundle By Name(cluster=w701, "Cal Log"=w683) -> (w700:T9)
                n459 = property on="Cal Table" class="Tbl (strict)"("Value"=w683) -> ()  [unwired: 2 in, 2 out]
              }
            }
          }
          frame True {
          }
        }
        n460 = Insert Into Array(array=w664, index=0, new element=w663) -> (w665:string[])
      }
      frame "Load Targets" {
        w767 = 0 ("length")
        # "#Change In \"A\" selection added selection of \"RIO\" that links 25A Targets and Setpoints"
        n461 = Unbundle By Name(w770) -> ("Cal Log"=w735:string[][], "Cal Targets Path"=w777:path, "Targets"=w772:T6, "Cal Target Array"=w757:string[], "Verify Table"=w724:string[][], "Channel to Cal"=w746:T1)
        n462 = property on="Cancel Verify" class="Bool"("DisabledEnum"=T10."Enabled" ("Disabled")) -> ()  [unwired: 2 in, 2 out]
        n463 = property on="Cal Table" class="Tbl (strict)"("Active Cell"=T12 {"Row"=-2, "Column"=-2} ("Active Cell:Active Cell"), "Cell BG Color"=u32 16448250) -> ()  [unwired: 2 in, 2 out]
        n464 = Index Array(array=w735, index (row)=w746) -> (element=w756:string[])  [unwired: 1 in]
        n465 = call <vilib>:"Open Config Data.vi"("configuration file path"=w777) -> ("error out"=w775:errorcluster, "refnum"=w776:T15)  [unwired: 8 in, 1 out]
        n466 = Array Subset "Calibration"(array=w756, index=2, length=10) -> (w719:string[])
        n467 = Array Subset "Verification"(array=w756, index=18, length=20) -> (w726:string[])
        n468 = property on="Apply Cal" class="Bool"("DisabledEnum"=T10."Disabled and Grayed Out" ("Disabled")) -> ()  [unwired: 2 in, 2 out]
        n469 = call <userlib>:"Read INI Cluster__ogtk.vi"("error in (no error)"=w775, "INI Fomatted Cluster Type"=w772, "refnum"=w776) -> ("error out"=w773:errorcluster, "INI Fomatted Cluster"=w771:variant, "dup refnum"=w774:T15)  [unwired: 4 in, 2 out]
        n470 = Index Array(array=w726, index #1=1 ("index"), index #2=3 ("index"), index #3=5 ("index"), index #4=7 ("index"), index #5=9 ("index")) -> (element #1=w745:string, element #2=w742:string, element #3=w744:string, element #4=w741:string, element #5=w743:string)
        n471 = call <vilib>:"Close Config Data.vi"("error in (no error)"=w773, "refnum"=w774) -> ()  [unwired: 8 in, 2 out]
        n472 = Fract/Exp String To Number(string=w719) -> (number=w729:dbl[])  [unwired: 3 in, 1 out]
        n473 = Empty Array?(array=w719) -> ()  [unwired: 1 out]
        n474 = Empty String/Path?(string/path=w745) -> (empty?=w738:bool)
        n475 = Empty String/Path?(string/path=w744) -> (empty?=w737:bool)
        n476 = Empty String/Path?(string/path=w743) -> (empty?=w736:bool)
        n477 = Variant To Data(type=w772, Variant=w771) -> (data=w760:T6)  [unwired: 1 in, 1 out]
        n478 = Index Array(array=w757, index=w746) -> (element=w761:string)
        n479 = Empty String/Path?(string/path=w742) -> (empty?=w740:bool)
        n480 = Empty String/Path?(string/path=w741) -> (empty?=w739:bool)
        n481 = Compound Arithmetic op=AND(w738, w740, w737, w739, w736) -> (w720:bool)
        n482 = case shown="\"DegC\"" w761 {
          tunnel: w760 -> [w825 w828 w831 w834 w837 w840]
          tunnel: [w823 w826 w829 w832 w835 w838] -> w758
          tunnel: [w824 w827 w830 w833 w836 w839] -> w759
          frame "V", Default {
            n483 = Unbundle By Name(w825) -> ("V Targets"=w824:T7, "V Setpoints"=w823:T8)
          }
          frame "A" {
            n484 = Unbundle By Name(w828) -> ("A Targets"=w827:T7, "A Setpoints"=w826:T8)
          }
          frame "DegC" {
            n485 = Unbundle By Name(w831) -> ("DegC Targets"=w830:T7, "DegC Setpoints"=w829:T8)
          }
          frame "kPa" {
            n486 = Unbundle By Name(w834) -> ("kPa Targets"=w833:T7, "kPa Setpoints"=w832:T8)
          }
          frame "LpH" {
            n487 = Unbundle By Name(w837) -> ("LpH Targets"=w836:T7, "LpH Setpoints"=w835:T8)
          }
          frame "CT" {
            n488 = Unbundle By Name(w840) -> ("CT Targets"=w839:T7, "CT Setpoints"=w838:T8)
          }
        }
        n489 = case shown="True" w720 {
          tunnel: w726 -> [_ w798]
          tunnel: w724 -> [w790 w797]
          tunnel: [w790 w791] -> w723
          frame True {
          }
          frame False {
            n490 = for {
              tunnel: w798 -> [w804] mode=indexing
              tunnel: [w804] -> w793 mode=indexing if=w800
              tunnel: [w804] -> w792 mode=indexing if=w799
              i -> [w803]
              n491 = Quotient & Remainder(x=w803, y=2) -> (x-y*floor(x/y)=w801:i32)  [unwired: 1 out]
              n492 = Equal To 0?(x=w801) -> (x = 0?=w800:bool)
              n493 = Not(x=w800) -> (.not. x?=w799:bool)
            }
            n494 = Replace Array Subset(array=w797, new element=w793, index (col)=0 ("disabled index (col)")) -> (w796:string[][])  [unwired: 1 in]
            n495 = Replace Array Subset(array=w796, new element=w792, index (col)=1 ("disabled index (col)")) -> (w791:string[][])  [unwired: 1 in]
          }
        }
        n496 = case shown="False" w720 {
          tunnel: w722 -> [w787 w789]
          tunnel: [w786 w789] -> w721
          frame False {
            n497 = Insert Into Array(array=w787, index=0, new element=string[] ["Calc Dev"]) -> (w786:string[])
          }
          frame True {
          }
        }
        n498 = for {
          tunnel: w719 -> [w784] mode=indexing
          tunnel: [w783] -> w718 mode=indexing
          n499 = Empty String/Path?(string/path=w784) -> (empty?=w783:bool)
        }
        n500 = Cluster To Array(cluster=w759) -> (array=w768:dbl[])
        n501 = Cluster To Array(cluster=w758) -> (array=w725:dbl[])
        n502 = And Array Elements(Boolean array=w718) -> (logical AND=w717:bool)
        n503 = Delete From Array(array=w768, length=w767, index=w767) -> (deleted portion=w763:dbl[], array with subset deleted=w766:dbl[])
        n504 = call-poly <userlib>:"Remove Duplicates from 1D Array__ogtk.vi"("Input Array"=w766) -> ("Output Array"=w765:dbl[])  [unwired: 1 out]
        n505 = Build Array (concatenate)(w763, w765) -> (w764:dbl[])
        n506 = Number To Fractional String(number=w764, precision (6)=i16 3) -> (F-format string=w769:string[])  [unwired: 2 in]
        n507 = case shown="False" w717 {
          tunnel: w725 -> [_ w822]
          tunnel: [w810 w821] -> w734
          tunnel: [w814 w820] -> w733
          tunnel: [w813 w819] -> w732
          tunnel: [w812 w818] -> w731
          tunnel: [w811 w817] -> w730
          tunnel: w729 -> [w815 _]
          tunnel: [w809 w816] -> w716
          tunnel: [w808 w816] -> w715
          tunnel: [w807 w816] -> w714
          tunnel: [w806 w816] -> w713
          tunnel: [w805 w816] -> w712
          frame False {
            n508 = Index Array(array=w815) -> (element #1=w809:dbl, element #2=w814:dbl, element #3=w808:dbl, element #4=w813:dbl, element #5=w807:dbl, element #6=w812:dbl, element #7=w806:dbl, element #8=w811:dbl, element #9=w805:dbl, element #10=w810:dbl)  [unwired: 10 in]
          }
          frame True {
            w816 = 0.0 ("Label")
            n509 = Index Array(array=w822) -> (element #1=w820:dbl, element #2=w819:dbl, element #3=w818:dbl, element #4=w817:dbl, element #5=w821:dbl)  [unwired: 5 in]
          }
        }
        n510 = Replace Array Subset(array=w724, new element=w769, index (col)=0 ("disabled index (col)")) -> (w728:string[][])  [unwired: 1 in]
        n511 = Select(t=w728, s=w720, f=w723) -> (s? t:f=w727:string[][])
        n512 = local write "Reading Value 1"(w716) -> ()
        n513 = local write "Reading Value 2"(w715) -> ()
        n514 = local write "Reading Value 3"(w714) -> ()
        n515 = local write "Reading Value 4"(w713) -> ()
        n516 = local write "Reading Value 5"(w712) -> ()
        n517 = local write "Cal Value 1"(w733) -> ()
        n518 = local write "Cal Value 2"(w732) -> ()
        n519 = local write "Cal Value 3"(w731) -> ()
        n520 = local write "Cal Value 4"(w730) -> ()
        n521 = local write "Cal Value 5"(w734) -> ()
        n522 = Bundle By Name(cluster=w770, "Targets"=w760, "Verify Table"=w727) -> (w779:T9)
        n523 = property on="Verify Table" class="Tbl (strict)"("Value"=w727) -> ()  [unwired: 2 in, 2 out]
      }
      frame "Start Cal" {
        w841 = T10."Disabled and Grayed Out" ("Disabled")
        w844 = T10."Enabled" ("Disabled")
        n524 = property on="Header" class="Bool"("DisabledEnum"=w841) -> ()  [unwired: 2 in, 2 out]
        n525 = property on="Channel to Cal" class="Enum (strict)"("DisabledEnum"=w841) -> ()  [unwired: 2 in, 2 out]
        n526 = property on="View Spreadsheet" class="Bool"("DisabledEnum"=w841) -> ()  [unwired: 2 in, 2 out]
        n527 = property on="Cal Tab" class="TabCtl (strict)"("Visible"=TRUE) -> ()  [unwired: 2 in, 2 out]
        n528 = property on="Start Cal" class="Bool"("DisabledEnum"=w841) -> ()  [unwired: 2 in, 2 out]
        n529 = disable-structure shown="Disabled" {
          disable-tunnel: w841 -> [w846 _]
          frame Disabled {
            n530 = property on="Cal Unit" class="Enum (strict)"("DisabledEnum"=w846) -> ()  [unwired: 2 in, 2 out]
          }
          frame Enabled {
          }
        }
        n531 = property on="Start Verification" class="Bool"("DisabledEnum"=w841) -> ()  [unwired: 2 in, 2 out]
        n532 = property on="Reading Value 1" class="DigNum (strict)"("DisabledEnum"=w844) -> ()  [unwired: 2 in, 2 out]
        n533 = property on="Cal Value 1" class="DigNum (strict)"("DisabledEnum"=w844) -> ()  [unwired: 2 in, 2 out]
        n534 = property on="1st Point Cal" class="Bool (strict)"("DisabledEnum"=w844) -> ()  [unwired: 2 in, 2 out]
        n535 = property on="Reading Value 2" class="DigNum (strict)"("DisabledEnum"=w844) -> ()  [unwired: 2 in, 2 out]
        n536 = property on="Cal Value 2" class="DigNum (strict)"("DisabledEnum"=w844) -> ()  [unwired: 2 in, 2 out]
        n537 = property on="2nd Point Cal" class="Bool (strict)"("DisabledEnum"=w844) -> ()  [unwired: 2 in, 2 out]
        n538 = property on="Reading Value 3" class="DigNum (strict)"("DisabledEnum"=w844) -> ()  [unwired: 2 in, 2 out]
        n539 = property on="Cal Value 3" class="DigNum (strict)"("DisabledEnum"=w844) -> ()  [unwired: 2 in, 2 out]
        n540 = property on="3rd Point Cal" class="Bool (strict)"("DisabledEnum"=w844) -> ()  [unwired: 2 in, 2 out]
        n541 = property on="Reading Value 4" class="DigNum (strict)"("DisabledEnum"=w844) -> ()  [unwired: 2 in, 2 out]
        n542 = property on="Cal Value 4" class="DigNum (strict)"("DisabledEnum"=w844) -> ()  [unwired: 2 in, 2 out]
        n543 = property on="4th Point Cal" class="Bool (strict)"("DisabledEnum"=w844) -> ()  [unwired: 2 in, 2 out]
        n544 = property on="Reading Value 5" class="DigNum (strict)"("DisabledEnum"=w844) -> ()  [unwired: 2 in, 2 out]
        n545 = property on="Cal Value 5" class="DigNum (strict)"("DisabledEnum"=w844) -> ()  [unwired: 2 in, 2 out]
        n546 = property on="5th Point Cal" class="Bool (strict)"("DisabledEnum"=w844) -> ()  [unwired: 2 in, 2 out]
      }
      frame "Calibrating 1".."Calibrating 6" {
        # "When it said \"Calibrating 1\"..\"Calibrating 5\" it was not accepting Calibrating 5"
        n547 = case shown="\"Calibrating 4\"" w852 {
          tunnel: [0.0 w858 w860 w862 w864 w866] -> w851
          tunnel: [1 1 2 3 4 5] -> w847
          frame Default {
          }
          frame "Calibrating 1" {
            n548 = local read "Cal Value 1"() -> (w858:dbl)
          }
          frame "Calibrating 2" {
            n549 = local read "Cal Value 2"() -> (w860:dbl)
          }
          frame "Calibrating 3" {
            n550 = local read "Cal Value 3"() -> (w862:dbl)
          }
          frame "Calibrating 4" {
            n551 = local read "Cal Value 4"() -> (w864:dbl)
          }
          frame "Calibrating 5" {
            n552 = local read "Cal Value 5"() -> (w866:dbl)
          }
        }
        n553 = property on="Cal Tab" class="TabCtl (strict)"("Visible"=TRUE) -> ()  [unwired: 2 in, 2 out]
        n554 = local write "Cal Tab"(enum32{"Apply", "Cal"}."Cal" ("Cal Tab")) -> ()
        n555 = local write "Master Value"(w851) -> ()
        n556 = Bundle By Name(cluster=w849, "LastCalPt"=w847) -> (w848:T9)
      }
      frame "Stop Calibrating" {
        n557 = local write "Cal Tab"(enum32{"Apply", "Cal"}."Apply" ("Cal Tab")) -> ()
      }
      frame "Calculate Coeffs" {
        w871 = T10."Enabled" ("Disabled")
        # "Used to enable and start the verification from here"
        n558 = Unbundle By Name(w878) -> ("Channel to Cal"=w874:T1, "Cal Unit"=w877:T2, "Verification"=w876:bool, "Cal Log"=w875:string[][])
        n559 = case shown="False" w876 {
          tunnel: [w892 w919] -> w883
          tunnel: [w891 w918] -> w882
          tunnel: [w890 w917] -> w881
          tunnel: w877 -> [w889 w916]
          tunnel: w875 -> [_ w920]
          tunnel: w874 -> [_ w921]
          tunnel: [w888 w915] -> w873
          tunnel: [w887 w914] -> w872
          frame False {
            n560 = case shown="\"V\", \"Hz\", Default" w889 {
              tunnel: [w909 w912] -> w892
              tunnel: [w908 1.0] -> w891
              tunnel: [w907 w912] -> w890
              tunnel: [w902 w912] -> w888
              tunnel: [w901 w912] -> w887
              frame "V", "Hz", Default {
                n561 = local read "Reading Value 1"() -> (w900:dbl)
                n562 = local read "Reading Value 2"() -> (w899:dbl)
                n563 = local read "Reading Value 3"() -> (w898:dbl)
                n564 = local read "Reading Value 4"() -> (w896:dbl)
                n565 = local read "Reading Value 5"() -> (w895:dbl)
                n566 = Build Array("Cal Value 1", "Cal Value 2", "Cal Value 3", "Cal Value 4", "Cal Value 5") -> (w906:dbl[])
                n567 = Build Array(w900, w899, w898, w896, w895) -> (w905:dbl[])
                n568 = call <vilib>:"General Polynomial Fit Coefficients.vi"("Y"=w906, "polynomial order"=4, "X"=w905) -> ("Polynomial Coefficients"=w904:dbl[])  [unwired: 11 in, 1 out]
                n569 = Index Array(array=w904) -> (element #1=w909:dbl, element #2=w908:dbl, element #3=w907:dbl, element #4=w902:dbl, element #5=w901:dbl)  [unwired: 5 in]
              }
              frame "deg C" {
                w912 = 0.0
              }
            }
          }
          frame True {
            n570 = case shown="Default" w916 {
              selector: w916 -> [w924 _]
              tunnel: w921 -> [w940 _]
              tunnel: w920 -> [w932 _]
              tunnel: [w927 w946] -> w919
              tunnel: [w926 1.0 ("Label")] -> w918
              tunnel: [w925 w946] -> w917
              tunnel: [w923 w946] -> w915
              tunnel: [w922 w946] -> w914
              frame Default {
                n571 = Format Into String(w940) -> (resulting string=w937:string)  [unwired: 3 in, 1 out]
                n572 = Format Into String(w924) -> (resulting string=w933:string)  [unwired: 3 in, 1 out]
                n573 = Index Array(array=w932, index (col) #1=0 ("disabled index (col)"), index (col) #2=1 ("index (col)")) -> (element #1=w938:string[], element #2=w934:string[])  [unwired: 2 in]
                n574 = call-poly <userlib>:"Search Array__ogtk.vi"("Array"=w938, "Element Data"=w937) -> ("Indices of Elements"=w935:i32[])  [unwired: 7 in]
                n575 = for {
                  tunnel: w935 -> [w941] mode=indexing
                  tunnel: w934 -> [w945]
                  tunnel: w933 -> [w943]
                  tunnel: [w941] -> w931
                  stop <- w942 stop-if-true
                  n576 = Index Array(array=w945, index=w941) -> (element=w944:string)
                  n577 = Equal?(x=w943, y=w944) -> (x = y?=w942:bool)
                }
                n578 = Index Array(array=w932, index (row)=w931) -> (element=w930:string[])  [unwired: 1 in]
                n579 = Fract/Exp String To Number(string=w930) -> (number=w929:dbl[])  [unwired: 3 in, 1 out]
                n580 = Index Array(array=w929, index #1=12 ("index")) -> (element #1=w927:dbl, element #2=w926:dbl, element #3=w925:dbl, element #4=w923:dbl, element #5=w922:dbl)  [unwired: 4 in]
              }
              frame "deg C" {
                w946 = 0.0 ("Label")
              }
            }
          }
        }
        "a0" <- w883
        "a2" <- w881
        "a1" <- w882
        "a4" <- w872
        "a3" <- w873
        n581 = property on="Cal Table" class="Tbl (strict)"("DisabledEnum"=T10."Disabled and Grayed Out" ("Disabled")) -> ()  [unwired: 2 in, 2 out]
        n582 = property on="Save Cal" class="Bool"("DisabledEnum"=T10."Enabled" ("Disabled")) -> ()  [unwired: 2 in, 2 out]
        n583 = Insert Into Array(array=w884, index=0, new element=string[] ["Save Calibration"]) -> (w885:string[])
        n584 = property on="a0" class="DigNum (strict)"("DisabledEnum"=w871) -> ()  [unwired: 2 in, 2 out]
        n585 = property on="a1" class="DigNum (strict)"("DisabledEnum"=w871) -> ()  [unwired: 2 in, 2 out]
        n586 = property on="a2" class="DigNum (strict)"("DisabledEnum"=w871) -> ()  [unwired: 2 in, 2 out]
        n587 = property on="a3" class="DigNum (strict)"("DisabledEnum"=w871) -> ()  [unwired: 2 in, 2 out]
        n588 = property on="a4" class="DigNum (strict)"("DisabledEnum"=w871) -> ()  [unwired: 2 in, 2 out]
      }
      frame "Cal Review Prep" {
        w953 = T10."Disabled and Grayed Out" ("Disabled")
        n589 = Unbundle By Name(w954) -> ("Desired System.ID"=w955:string)
        n590 = Format Into String(format string="ni.var.psp://10.30.189.%s/Streaming Control/StreamCalibrated", w955) -> (resulting string=w963:string, error out=w964:errorcluster)  [unwired: 2 in]
        n591 = property on="Cal Tab" class="TabCtl (strict)"("Visible"=FALSE) -> ()  [unwired: 2 in, 2 out]
        n592 = property on="Verify Tab" class="TabCtl (strict)"("Visible"=TRUE) -> (error out=w950:errorcluster)  [unwired: 2 in, 1 out]
        n593 = shared-variable-open(w963, w964, FALSE) -> (w957:refnum<k21>, w960:errorcluster)  [unwired: 1 in]
        n594 = shared-variable-write(w957, w960, TRUE ("data in")) -> (w958:refnum<k21>, w959:errorcluster)
        n595 = property on="Verify Table" class="Tbl (strict)"(error in=w950, "Key Focus"=TRUE, "EditPos"=T12 {"Row"=0, "Column"=1} ("Active Cell:Active Cell")) -> ()  [unwired: 1 in, 2 out]
        n596 = Close Variable Connection(8:w959, 11:w958) -> ()  [unwired: 1 out]
        n597 = Insert Into Array(array=w968, index=0, new element=string[] ["Cal Review"]) -> (w967:string[])
        n598 = property on="Reading Value 1" class="DigNum (strict)"("DisabledEnum"=w953) -> ()  [unwired: 2 in, 2 out]
        n599 = property on="Cal Value 1" class="DigNum (strict)"("DisabledEnum"=w953) -> ()  [unwired: 2 in, 2 out]
        n600 = property on="1st Point Cal" class="Bool (strict)"("DisabledEnum"=w953) -> ()  [unwired: 2 in, 2 out]
        n601 = property on="Reading Value 2" class="DigNum (strict)"("DisabledEnum"=w953) -> ()  [unwired: 2 in, 2 out]
        n602 = property on="Cal Value 2" class="DigNum (strict)"("DisabledEnum"=w953) -> ()  [unwired: 2 in, 2 out]
        n603 = property on="2nd Point Cal" class="Bool (strict)"("DisabledEnum"=w953) -> ()  [unwired: 2 in, 2 out]
        n604 = property on="Reading Value 3" class="DigNum (strict)"("DisabledEnum"=w953) -> ()  [unwired: 2 in, 2 out]
        n605 = property on="Cal Value 3" class="DigNum (strict)"("DisabledEnum"=w953) -> ()  [unwired: 2 in, 2 out]
        n606 = property on="3rd Point Cal" class="Bool (strict)"("DisabledEnum"=w953) -> ()  [unwired: 2 in, 2 out]
        n607 = property on="Reading Value 4" class="DigNum (strict)"("DisabledEnum"=w953) -> ()  [unwired: 2 in, 2 out]
        n608 = property on="Cal Value 4" class="DigNum (strict)"("DisabledEnum"=w953) -> ()  [unwired: 2 in, 2 out]
        n609 = property on="4th Point Cal" class="Bool (strict)"("DisabledEnum"=w953) -> ()  [unwired: 2 in, 2 out]
        n610 = property on="Reading Value 5" class="DigNum (strict)"("DisabledEnum"=w953) -> ()  [unwired: 2 in, 2 out]
        n611 = property on="Cal Value 5" class="DigNum (strict)"("DisabledEnum"=w953) -> ()  [unwired: 2 in, 2 out]
        n612 = property on="5th Point Cal" class="Bool (strict)"("DisabledEnum"=w953) -> ()  [unwired: 2 in, 2 out]
      }
      frame "Cal Review" {
        n613 = Unbundle By Name(w979) -> ("Auto"=w977:bool, "Verify Table"=w980:string[][])
        n614 = property on="Verify Table" class="Tbl (strict)"() -> ("EditPos"=w993:T12)  [unwired: 2 in, 2 out]
        n615 = Unbundle(w993) -> ("Row"=w991:i32)  [unwired: 1 out]
        n616 = local read "Ver Reading"() -> (w970:dbl)
        n617 = Greater Or Equal To 0?(x=w991) -> (x >= 0?=w992:bool)
        n618 = Index Array(array=w980, index (row)=w991, index (col)=0 ("disabled index (col)")) -> (element=w983:string)
        n619 = Fract/Exp String To Number(string=w983) -> (number=w972:dbl)  [unwired: 3 in, 1 out]
        n620 = case shown="True" w992 {
          tunnel: w991 -> [_ w1001]
          frame False {
          }
          frame True {
            "Row" <- w1001
          }
        }
        n621 = Increment(x=w970) -> (x+1=w984:dbl)
        n622 = Increment(x=w972) -> (x+1=w985:dbl)
        n623 = Subtract(x=w984, y=w985) -> (x-y=w973:dbl)
        n624 = Divide(x=w973, y=w984) -> (x/y=w989:dbl)
        n625 = local read "Lost Connection"() -> (w969:bool)
        n626 = Empty String/Path?(string/path=w983) -> (empty?=w976:bool)
        n627 = Absolute Value(x=w989) -> (abs(x)=w971:dbl)
        n628 = Not(x=w976) -> (.not. x?=w986:bool)
        n629 = Less?(x=w971, y=0.1) -> (x < y?=w987:bool)
        n630 = Compound Arithmetic op=AND(w977, w987, w986) -> (w982:bool)
        n631 = call "Reading Delay.vi"("Delay"="ms", "In Range"=w982) -> ("Take Reading"=w975:bool)  [unwired: 9 in]
        n632 = case shown="False" w969 {
          tunnel: [string[] ["Main", "Cal Review"] string[] ["End Cal"]] -> w997
          frame False {
          }
          frame True {
          }
        }
        n633 = case shown="True" w975 {
          selector: w975 -> [_ w1000]
          frame False {
          }
          frame True {
            n634 = property on="Verify Read" class="Bool (strict)"("Val(Sgnl)"=w1000) -> ()  [unwired: 2 in, 2 out]
          }
        }
        n635 = Bundle By Name(cluster=w979, "Init Mean"=FALSE) -> (w974:T9)
        n636 = Insert Into Array(array=w995, index=0, new element=w997) -> (w996:string[])
      }
      frame "Stop Verification" {
        w1002 = T10."Enabled" ("Disabled")
        n637 = property on="Header" class="Bool"("DisabledEnum"=w1002) -> ()  [unwired: 2 in, 2 out]
        n638 = property on="Channel to Cal" class="Enum (strict)"("DisabledEnum"=w1002) -> ()  [unwired: 2 in, 2 out]
        n639 = property on="View Spreadsheet" class="Bool"("DisabledEnum"=w1002) -> ()  [unwired: 2 in, 2 out]
        n640 = property on="Cal Unit" class="Enum (strict)"("DisabledEnum"=T10."Enabled" ("Disabled")) -> ()  [unwired: 2 in, 2 out]
        n641 = property on="Start Cal" class="Bool"("DisabledEnum"=w1002) -> ()  [unwired: 2 in, 2 out]
        n642 = disable-structure shown="Disabled" {
          disable-tunnel: w1002 -> [w1007 _]
          frame Disabled {
            n643 = property on="Start Verification" class="Bool"("DisabledEnum"=w1007) -> ()  [unwired: 2 in, 2 out]
          }
          frame Enabled {
          }
        }
        n644 = property on="Verify Tab" class="TabCtl (strict)"("Visible"=FALSE) -> ()  [unwired: 2 in, 2 out]
      }
      frame "Save Cal" {
        w1054 = u16 4 ("y")
        n645 = Unbundle By Name(w1029) -> ("Cal File Path"=w1039:path, "Cal Log Header"=w1061:string[], "Cal Log"=w1025:string[][], "Channel to Cal"=w1037:T1, "Cal Unit"=w1038:T2, "Verification"=w1028:bool, "Verify Table"=w1040:string[][])
        n646 = local read "Reading Value 1"() -> (w1022:dbl)
        n647 = local read "Reading Value 2"() -> (w1020:dbl)
        n648 = local read "Reading Value 3"() -> (w1018:dbl)
        n649 = local read "Reading Value 4"() -> (w1016:dbl)
        n650 = local read "Reading Value 5"() -> (w1014:dbl)
        n651 = local read "Cal Value 1"() -> (w1021:dbl)
        n652 = local read "Cal Value 2"() -> (w1019:dbl)
        n653 = local read "Cal Value 3"() -> (w1017:dbl)
        n654 = local read "Cal Value 4"() -> (w1015:dbl)
        n655 = local read "Cal Value 5"() -> (w1013:dbl)
        n656 = local read "a0"() -> (w1012:dbl)
        n657 = local read "a1"() -> (w1011:dbl)
        n658 = local read "a2"() -> (w1010:dbl)
        n659 = local read "a3"() -> (w1009:dbl)
        n660 = local read "a4"() -> (w1008:dbl)
        n661 = Build Array(w1022, w1021, w1020, w1019, w1018, w1017, w1016, w1015, w1014, w1013, w1012, w1011, w1010, w1009, w1008) -> (w1067:dbl[])
        n662 = Format Into String(w1037) -> (resulting string=w1033:string)  [unwired: 3 in, 1 out]
        n663 = Format Into String(w1038) -> (resulting string=w1030:string)  [unwired: 3 in, 1 out]
        n664 = Index Array(array=w1025, index (col) #1=0 ("disabled index (col)"), index (col) #2=1 ("index (col)")) -> (element #1=w1034:string[], element #2=w1032:string[])  [unwired: 2 in]
        n665 = Search 1D Array(1D array=w1034, element=w1033) -> (index of element=w1031:i32)  [unwired: 1 in]
        n666 = disable-structure shown="Disabled" {
          disable-tunnel: w1032 -> [w1074 _]
          disable-tunnel: w1031 -> [w1073 w1075]
          disable-tunnel: w1030 -> [w1072 _]
          disable-tunnel: [w1071 w1075] -> w1024
          frame Disabled {
            n667 = Search 1D Array(1D array=w1074, element=w1072, start index (0)=w1073) -> (index of element=w1071:i32)
          }
          frame Enabled {
          }
        }
        n668 = Index Array(array=w1040, index (col) #1=0 ("disabled index (col)"), index (col) #2=1 ("disabled index (col)")) -> (element #1=w1044:string[], element #2=w1043:string[])  [unwired: 2 in]
        n669 = Format Date/Time String(time format string (%c)="%d%b%y %I:%M:%S %p") -> (date/time string=w1065:string)  [unwired: 2 in]
        n670 = Interleave 1D Arrays(w1044, w1043) -> (w1042:string[])
        n671 = Index Array(array=w1025, index (row)=w1024) -> (element=w1023:string[])  [unwired: 1 in]
        n672 = To Upper Case(1:w1065) -> (0:w1027:string)
        n673 = case shown="False" w1028 {
          tunnel: w1067 -> [w1079 _]
          tunnel: [w1077 w1081] -> w1066
          tunnel: [w1076 w1080] -> w1026
          tunnel: w1027 -> [w1076 _]
          tunnel: w1023 -> [_ w1083]
          frame False {
            n674 = Number To Fractional String(number=w1079, precision (6)=i16 16) -> (F-format string=w1077:string[])  [unwired: 2 in]
          }
          frame True {
            n675 = Array Subset(array=w1083, index=2, length=9) -> (w1081:string[])
            n676 = Index Array(array=w1083, index=11) -> (element=w1080:string)
          }
        }
        n677 = Build Array (concatenate)(w1033, w1030, w1066, w1026, w1042) -> (w1063:string[])
        n678 = Greater?(x=w1024, y=w1054) -> (0:w1053:bool)
        n679 = Subtract(x=w1024, y=w1054) -> (x-y=w1052:i32)
        n680 = Bundle(cluster=T12 {"Row"=0, "Column"=0} ("Active Cell:Active Cell"), "Row"=w1024, "Column"=-2) -> (w1055:T12)
        n681 = Select(t=w1052, s=w1053, f=u16 0 ("y")) -> (s? t:f=w1049:i32)
        n682 = Replace Array Subset(array=w1025, new element=w1063, index (row)=w1024) -> (w1060:string[][])  [unwired: 1 in]
        n683 = Bundle(cluster=T12 {"Row"=0, "Column"=0} ("Active Cell:Active Cell"), "Row"=w1049, "Column"=0) -> (w1048:T12)
        n684 = Build Array (concatenate)(w1061, w1060) -> (w1059:string[][])
        n685 = Insert Into Array(array=w1068, index=0, new element=string[] ["Write to Excel", "Load Cal File", "End Cal", "Increment Channel"]) -> (w1069:string[])
        n686 = property on="Cal Table" class="Tbl (strict)"("Active Cell"=w1055, "Cell BG Color"=u32 16775793, "Index Values"=w1048) -> ()  [unwired: 2 in, 2 out]
        n687 = call-poly <vilib>:"Write To Spreadsheet File.vi"("delimiter (\\t)"="," ("delimiter (\\t)"), "2D data"=w1059, "file path (dialog if empty)"=w1039) -> ()  [unwired: 5 in, 1 out]
      }
      frame "Save Calibration" {
        w1132 = u16 4 ("y")
        n688 = Unbundle By Name(w1107) -> ("Cal File Path"=w1117:path, "Cal Log Header"=w1139:string[], "Cal Log"=w1103:string[][], "Channel to Cal"=w1115:T1, "Cal Unit"=w1116:T2, "Verification"=w1106:bool, "Verify Table"=w1118:string[][])
        n689 = local read "Reading Value 1"() -> (w1100:dbl)
        n690 = local read "Reading Value 2"() -> (w1098:dbl)
        n691 = local read "Reading Value 3"() -> (w1096:dbl)
        n692 = local read "Reading Value 4"() -> (w1094:dbl)
        n693 = local read "Reading Value 5"() -> (w1092:dbl)
        n694 = local read "Cal Value 1"() -> (w1099:dbl)
        n695 = local read "Cal Value 2"() -> (w1097:dbl)
        n696 = local read "Cal Value 3"() -> (w1095:dbl)
        n697 = local read "Cal Value 4"() -> (w1093:dbl)
        n698 = local read "Cal Value 5"() -> (w1091:dbl)
        n699 = local read "a0"() -> (w1090:dbl)
        n700 = local read "a1"() -> (w1089:dbl)
        n701 = local read "a2"() -> (w1088:dbl)
        n702 = local read "a3"() -> (w1087:dbl)
        n703 = local read "a4"() -> (w1086:dbl)
        n704 = Build Array(w1100, w1099, w1098, w1097, w1096, w1095, w1094, w1093, w1092, w1091, w1090, w1089, w1088, w1087, w1086) -> (w1145:dbl[])
        n705 = Format Into String(w1115) -> (resulting string=w1111:string)  [unwired: 3 in, 1 out]
        n706 = Format Into String(w1116) -> (resulting string=w1108:string)  [unwired: 3 in, 1 out]
        n707 = Index Array(array=w1103, index (col) #1=0 ("disabled index (col)"), index (col) #2=1 ("index (col)")) -> (element #1=w1112:string[], element #2=w1110:string[])  [unwired: 2 in]
        n708 = Search 1D Array(1D array=w1112, element=w1111) -> (index of element=w1109:i32)  [unwired: 1 in]
        n709 = disable-structure shown="Enabled" {
          disable-tunnel: w1110 -> [w1152 _]
          disable-tunnel: w1109 -> [w1151 w1153]
          disable-tunnel: w1108 -> [w1150 _]
          disable-tunnel: [w1149 w1153] -> w1102
          frame Disabled {
            n710 = Search 1D Array(1D array=w1152, element=w1150, start index (0)=w1151) -> (index of element=w1149:i32)
          }
          frame Enabled {
          }
        }
        n711 = Index Array(array=w1118, index (col) #1=0 ("disabled index (col)"), index (col) #2=1 ("disabled index (col)")) -> (element #1=w1122:string[], element #2=w1121:string[])  [unwired: 2 in]
        n712 = Format Date/Time String(time format string (%c)="%d%b%y %I:%M:%S %p") -> (date/time string=w1143:string)  [unwired: 2 in]
        n713 = Interleave 1D Arrays(w1122, w1121) -> (w1120:string[])
        n714 = Index Array(array=w1103, index (row)=w1102) -> (element=w1101:string[])  [unwired: 1 in]
        n715 = To Upper Case(1:w1143) -> (0:w1105:string)
        n716 = case shown="False" w1106 {
          tunnel: w1145 -> [w1157 _]
          tunnel: [w1155 w1159] -> w1144
          tunnel: [w1154 w1158] -> w1104
          tunnel: w1105 -> [w1154 _]
          tunnel: w1101 -> [_ w1161]
          frame False {
            n717 = Number To Fractional String(number=w1157, precision (6)=i16 16) -> (F-format string=w1155:string[])  [unwired: 2 in]
          }
          frame True {
            n718 = Array Subset(array=w1161, index=2, length=9) -> (w1159:string[])
            n719 = Index Array(array=w1161, index=11) -> (element=w1158:string)
          }
        }
        n720 = Build Array (concatenate)(w1111, w1108, w1144, w1104, w1120) -> (w1141:string[])
        n721 = Greater?(x=w1102, y=w1132) -> (0:w1131:bool)
        n722 = Subtract(x=w1102, y=w1132) -> (x-y=w1130:i32)
        n723 = Bundle(cluster=T12 {"Row"=0, "Column"=0} ("Active Cell:Active Cell"), "Row"=w1102, "Column"=-2) -> (w1133:T12)
        n724 = Select(t=w1130, s=w1131, f=u16 0 ("y")) -> (s? t:f=w1127:i32)
        n725 = Replace Array Subset(array=w1103, new element=w1141, index (row)=w1102) -> (w1138:string[][])  [unwired: 1 in]
        n726 = Bundle(cluster=T12 {"Row"=0, "Column"=0} ("Active Cell:Active Cell"), "Row"=w1127, "Column"=0) -> (w1126:T12)
        n727 = Build Array (concatenate)(w1139, w1138) -> (w1137:string[][])
        n728 = Insert Into Array(array=w1146, index=0, new element=string[] ["Write to Excel", "Load Cal File", "Cal Review Prep"]) -> (w1147:string[])
        n729 = property on="Cal Table" class="Tbl (strict)"("Active Cell"=w1133, "Cell BG Color"=u32 16775793, "Index Values"=w1126) -> ()  [unwired: 2 in, 2 out]
        n730 = call-poly <vilib>:"Write To Spreadsheet File.vi"("delimiter (\\t)"="," ("delimiter (\\t)"), "2D data"=w1137, "file path (dialog if empty)"=w1117) -> ()  [unwired: 5 in, 1 out]
      }
      frame "Distribute Calibration" {
        # "have to add in waiting screen, reread on main program, switch to streaming calibrated data and verification for that"
        n731 = Unbundle By Name(w1168) -> ("Desired System.ID"=w1165:string, "Cal File Path"=w1170:path)
        n732 = Concatenate Strings("10.30.189." ("string"), w1165) -> (w1166:string)
        n733 = Format Into String(format string="%s.cal", w1165) -> (resulting string=w1167:string)  [unwired: 2 in, 1 out]
        n734 = flat-sequence {
          tunnel: w1166 -> [w1176]
          tunnel: w1167 -> [w1175]
          tunnel: w1170 -> [w1174]
          frame #0 {
            n735 = call <vilib>:"FTP Put File.vi"("password"="", "user"="anonymous", "local path"=w1174, "remote path"=w1175, "host"=w1176) -> ()  [unwired: 5 in, 2 out]
          }
        }
      }
      frame "Calc Dev" {
        n736 = Unbundle By Name(w1184) -> ("Verify Table"=w1181:string[][], "Cal Unit"=w1179:T2, "Rack Version"=w1178:T5, "Verify Table Ref"=w1177:refnum<vi>)
        n737 = call "Calc Dev (DAQ Rack).vi"("Verify Table IN"=w1181, "Units"=w1179, "Rack Version"=w1178, "Dev Table 1 Ref"=w1177) -> ("Verify Table OUT"=w1180:string[][])  [unwired: 15 in]
        n738 = local write "Verify Table"(w1180) -> ()
        n739 = Bundle By Name(cluster=w1184, "Verify Table"=w1180) -> (w1183:T9)
        n740 = Insert Into Array(array=w1186, index=0, new element=string[] []) -> (w1185:string[])
      }
      frame "Write to Excel" {
        n741 = Unbundle By Name(w1195) -> ("Cal Spreadsheet Path"=w1199:path, "Verify Table"=w1192:string[][], "Channel to Cal"=w1189:T1, "Cal Unit"=w1188:T2)
        n742 = flat-sequence {
          tunnel: w1199 -> [w1206]
          tunnel: [w1206] -> w1200
          tunnel: [w1203] -> w1193
          tunnel: w1192 -> [w1203]
          tunnel: [w1202] -> w1191
          tunnel: w1189 -> [w1202]
          tunnel: [w1201] -> w1190
          tunnel: w1188 -> [w1201]
          tunnel: w1200 -> [w1210]
          tunnel: w1193 -> [w1209]
          tunnel: w1191 -> [w1208]
          tunnel: w1190 -> [w1207]
          frame #0 {
            n743 = property on="Main Tab" class="TabCtl (strict)"("DisabledEnum"=T10."Disabled" ("Disabled")) -> ()  [unwired: 2 in, 2 out]
            n744 = property on="Load Indicator Tab" class="TabCtl (strict)"("Visible"=TRUE) -> ()  [unwired: 2 in, 2 out]
          }
          frame #1 {
            n745 = call "Gas Rack Write Data.vi"("Cal Unit"=w1207, "Channel to Cal"=w1208, "Verify Table"=w1209, "Cal Path"=w1210) -> ()  [unwired: 8 in]
          }
          frame #2 {
            n746 = property on="Main Tab" class="TabCtl (strict)"("DisabledEnum"=T10."Enabled" ("Disabled")) -> ()  [unwired: 2 in, 2 out]
            n747 = property on="Load Indicator Tab" class="TabCtl (strict)"("Visible"=FALSE) -> ()  [unwired: 2 in, 2 out]
          }
        }
        n748 = Insert Into Array(array=w1197, index=0, new element=string[] ["Recolor Tables"]) -> (w1196:string[])
      }
      frame "Recolor Tables" {
        n749 = Unbundle By Name(w1217) -> ("Verify Table Ref"=w1216:refnum<vi>)
        n750 = property on="Property Node" class="Tbl (strict)"(reference=w1216, "Active Cell"=T12 {"Row"=-2, "Column"=-2} ("Active Cell:Active Cell"), "Cell BG Color"=u32 15527148) -> (reference out=w1213:refnum<vi>)  [unwired: 1 in, 1 out]
        n751 = property on="Property Node" class="Tbl (strict)"(reference=w1213, "Active Cell"=T12 {"Row"=-2, "Column"=1} ("Active Cell:Active Cell"), "Cell BG Color"=u32 16448250) -> ()  [unwired: 1 in, 2 out]
      }
      frame "End Cal" {
        w1221 = FALSE ("1st Point Cal")
        w1224 = T10."Disabled and Grayed Out" ("Disabled")
        w1226 = 0.0 ("Reading Value 1")
        w1230 = FALSE ("Visible")
        n752 = disable-structure shown="Disabled" {
          frame Disabled {
            n753 = property on="Cancel Verify" class="Bool"("Value"=FALSE ("Cancel Cal")) -> ()  [unwired: 2 in, 2 out]
          }
          frame Enabled {
          }
        }
        n754 = property on="Output Tab" class="TabCtl (strict)"("Visible"=w1230) -> ()  [unwired: 2 in, 2 out]
        n755 = property on="Header Tab" class="TabCtl (strict)"("Visible"=w1230) -> ()  [unwired: 2 in, 2 out]
        n756 = property on="Load Indicator Tab" class="TabCtl (strict)"("Visible"=w1230) -> ()  [unwired: 2 in, 2 out]
        n757 = property on="Main Tab" class="TabCtl (strict)"("DisabledEnum"=T10."Enabled" ("Disabled")) -> ()  [unwired: 2 in, 2 out]
        n758 = property on="Header" class="Bool"("DisabledEnum"=T10."Enabled" ("Disabled")) -> ()  [unwired: 2 in, 2 out]
        n759 = local write "Reading Value 1"(w1226) -> ()
        n760 = local write "Cal Value 1"(w1226) -> ()
        n761 = local write "Reading Value 2"(w1226) -> ()
        n762 = local write "Cal Value 2"(w1226) -> ()
        n763 = local write "Reading Value 3"(w1226) -> ()
        n764 = local write "Cal Value 3"(w1226) -> ()
        n765 = local write "Reading Value 4"(w1226) -> ()
        n766 = local write "Cal Value 4"(w1226) -> ()
        n767 = local write "Reading Value 5"(w1226) -> ()
        n768 = local write "Cal Value 5"(w1226) -> ()
        n769 = local write "a0"(w1226) -> ()
        n770 = local write "a1"(w1226) -> ()
        n771 = local write "a2"(w1226) -> ()
        n772 = local write "a3"(w1226) -> ()
        n773 = local write "a4"(w1226) -> ()
        n774 = property on="Start Cal" class="Bool"("DisabledEnum"=w1224) -> ()  [unwired: 2 in, 2 out]
        n775 = property on="Channel to Cal" class="Enum (strict)"("DisabledEnum"=w1224) -> ()  [unwired: 2 in, 2 out]
        n776 = property on="View Spreadsheet" class="Bool"("DisabledEnum"=w1224) -> ()  [unwired: 2 in, 2 out]
        n777 = property on="Start Verification" class="Bool"("DisabledEnum"=w1224) -> ()  [unwired: 2 in, 2 out]
        n778 = local write "Tank IP:"("" ("Tank IP:")) -> ()
        n779 = local write "RIO Found"(FALSE ("RIO Found")) -> ()
        n780 = call "TCP Data Stream PC.vi"("Mode"=TCP_Data_Stream_Mode_(PC)."Close") -> ()  [unwired: 15 in, 4 out]
        n781 = disable-structure shown="Disabled" {
          disable-tunnel: w1224 -> [w1235 _]
          frame Disabled {
            n782 = property on="Cal Unit" class="Enum (strict)"("DisabledEnum"=w1235) -> ()  [unwired: 2 in, 2 out]
          }
          frame Enabled {
          }
        }
        n783 = local write "1st Point Cal"(w1221) -> ()
        n784 = local write "2nd Point Cal"(w1221) -> ()
        n785 = local write "3rd Point Cal"(w1221) -> ()
        n786 = local write "4th Point Cal"(w1221) -> ()
        n787 = local write "5th Point Cal"(w1221) -> ()
        n788 = Insert Into Array(array=w1233, index=0, new element=string[] ["Recolor Tables", "Init Cal"]) -> (w1234:string[])
      }
      frame "Increment Channel" {
        n789 = Unbundle By Name(w1239) -> ("Channel to Cal"=w1238:T1)
        n790 = Increment(x=w1238) -> (x+1=w1237:T1)
        n791 = Bundle By Name(cluster=w1239, "Channel to Cal"=w1237) -> (w1240:T9)
        n792 = local write "Channel to Cal"(w1237) -> ()
      }
      frame "Exit" {
        n793 = local write "Stop Second Loop"(TRUE ("Stop Second Loop")) -> ()
      }
    }
  }
  n794 = while {
    tunnel: w2 -> [_]
    shift-right: [w1246] -> _
    shift-left: _ -> [w1247]
    stop <- "Stop Second Loop" stop-if-true
    n795 = local read "Channel to Cal"() -> (w1245:T1)
    n796 = local read "RIO Found"() -> (w1250:bool)
    n797 = Wait (ms)(milliseconds to wait=u32 10) -> ()  [unwired: 1 out]
    n798 = case shown="True" w1250 {
      tunnel: w1245 -> [_ w1255]
      tunnel: [0.0 ("Data Out") w1257] -> w1246
      tunnel: w1247 -> [_ w1256]
      frame False {
      }
      frame True {
        n799 = call "Gas Rack AI Read.vi"("Channel to Cal"=w1255) -> ("Lost Connection"=→"Lost Connection":bool, "Available?"=w1253:bool, "Data"=w1254:dbl)  [unwired: 8 in]
        n800 = case shown="False" w1253 {
          tunnel: w1254 -> [_ w1260]
          tunnel: [w1258 w1259] -> w1257
          tunnel: w1256 -> [w1258 _]
          frame False {
          }
          frame True {
            n801 = call <vilib>:"Mean PtByPt.vi"("x"=w1260, "sample length"="avg") -> ("mean"=w1259:dbl)  [unwired: 2 in, 1 out]
          }
        }
      }
    }
    "Cal Reading" <- w1246
    "Ver Reading" <- w1246
  }
  n802 = disable-structure shown="Disabled" {
    frame Disabled {
      n803 = property on="Verify Tab" class="TabCtl (strict)"("Visible"=TRUE) -> (error out=w1263:errorcluster)  [unwired: 2 in, 1 out]
      n804 = property on="Verify Table" class="Tbl (strict)"(error in=w1263, "Key Focus"=TRUE, "EditPos"=T12 {"Row"=0, "Column"=1} ("Active Cell:Active Cell")) -> ()  [unwired: 1 in, 2 out]
    }
    frame Enabled {
    }
  }
  n805 = disable-structure shown="Disabled" {
    frame Disabled {
      w1287 = 0 ("length")
      # "#Change In \"A\" selection added selection of \"RIO\" that links 25A Targets and Setpoints"
      n806 = Unbundle By Name() -> (w1283:T17, "Cal Targets Path"=w1276, "Targets"=w1281, "Cal Target Array"=w1297, "Channel to Cal"=w1298, "Verify Table"=w1270)
      n807 = property on="Cancel Verify" class="Bool"("DisabledEnum"=T10."Enabled" ("Disabled")) -> ()  [unwired: 2 in, 2 out]
      n808 = property on="Cal Table" class="Tbl (strict)"("Active Cell"=T12 {"Row"=-2, "Column"=-2} ("Active Cell:Active Cell"), "Cell BG Color"=u32 16448250) -> ()  [unwired: 2 in, 2 out]
      n809 = call <vilib>:"Open Config Data.vi"("configuration file path"=w1276) -> ("error out"=w1278:errorcluster, "refnum"=w1277:T15)  [unwired: 8 in, 1 out]
      n810 = call <userlib>:"Read INI Cluster__ogtk.vi"("error in (no error)"=w1278, "INI Fomatted Cluster Type"=w1281, "refnum"=w1277) -> ("error out"=w1280:errorcluster, "INI Fomatted Cluster"=w1282:variant, "dup refnum"=w1279:T15)  [unwired: 4 in, 2 out]
      n811 = Index Array(array=w1297, index=w1298) -> (element=w1293)
      n812 = call <vilib>:"Close Config Data.vi"("error in (no error)"=w1280, "refnum"=w1279) -> ()  [unwired: 8 in, 2 out]
      n813 = Variant To Data(type=w1281, Variant=w1282) -> (data=w1294)  [unwired: 1 in, 1 out]
      n814 = case shown="\"V\", Default" w1293 {
        tunnel: w1294 -> [w1303 w1306 w1309 w1312 w1315 w1318]
        tunnel: [w1301 w1304 w1307 w1310 w1313 w1316] -> w1296
        tunnel: [w1302 w1305 w1308 w1311 w1314 w1317] -> w1295
        frame "V", Default {
          n815 = Unbundle By Name(w1303) -> ("V Targets"=w1302, "V Setpoints"=w1301)
        }
        frame "A" {
          n816 = Unbundle By Name(w1306) -> ("A Targets"=w1305, "A Setpoints"=w1304)
        }
        frame "DegC" {
          n817 = Unbundle By Name(w1309) -> ("DegC Targets"=w1308, "DegC Setpoints"=w1307)
        }
        frame "kPa" {
          n818 = Unbundle By Name(w1312) -> ("kPa Targets"=w1311, "kPa Setpoints"=w1310)
        }
        frame "LpH" {
          n819 = Unbundle By Name(w1315) -> ("LpH Targets"=w1314, "LpH Setpoints"=w1313)
        }
        frame "CT" {
          n820 = Unbundle By Name(w1318) -> ("CT Targets"=w1317, "CT Setpoints"=w1316)
        }
      }
      n821 = Cluster To Array(cluster=w1295) -> (array=w1286:void[])
      n822 = Cluster To Array(cluster=w1296) -> (array=w1285:void[])
      n823 = Delete From Array(array=w1286, length=w1287, index=w1287) -> (deleted portion=w1291, array with subset deleted=w1288)
      n824 = call-poly <userlib>:"Remove Duplicates from 1D Array__ogtk.vi"("Input Array"=w1288) -> ("Output Array"=w1289:dbl[])  [unwired: 1 out]
      n825 = Build Array (concatenate)(w1291, w1289) -> (w1290:dbl[])
      n826 = Number To Fractional String(number=w1290, precision (6)=i16 3) -> (F-format string=w1284:string[])  [unwired: 2 in]
      n827 = Index Array(array=w1285) -> (element #1=w1273, element #2=w1274, element #3=w1275, element #4=w1299, element #5=w1300)  [unwired: 5 in]
      n828 = Replace Array Subset(array=w1270, new element=w1284, index (col)=0 ("disabled index (col)")) -> (w1272:string[])  [unwired: 1 in]
      n829 = local write "Cal Value 1"(w1273) -> ()
      n830 = local write "Cal Value 2"(w1274) -> ()
      n831 = local write "Cal Value 3"(w1275) -> ()
      n832 = local write "Cal Value 4"(w1299) -> ()
      n833 = local write "Cal Value 5"(w1300) -> ()
      n834 = Bundle By Name(cluster=w1283, "Targets"=w1294, "Verify Table"=w1272) -> (w1269:cluster{})
      n835 = property on="Verify Table" class="Tbl (strict)"("Value"=w1272) -> ()  [unwired: 2 in, 2 out]
    }
    frame Enabled {
    }
  }
